vi "obs2lane2.vi"(11 "sensors inputs":dbl[][](array[numeric])=[[-2.6493086559458767, 9.313377271515247, 0.316177936945349, -1.2], [-2.6066100840450477, 9.354542103994737, 0.3157590885476819, -1.2], [-2.579340659822815, 9.43207739327695, 0.31450254335468053, -1.2], [-2.6132527619437576, 9.439068677849818, 0.5859163050429868, 1.2000000000000006], [-2.6655003955140795, 9.41719146151926, 0.4953083793337705, 0.40000000000000013], [-2.8189313467074544, 9.344249551531279, 0.5859163050429868, 1.2000000000000006], [-2.5692189092921667, 9.480018973387281, 0.5863351534406539, 1.2000000000000006], [-2.6731933264342116, 9.434269134901442, 0.5863351534406539, 1.2000000000000006], [-2.77635346299322, 9.386711660550553, 0.5863351534406539, 1.2000000000000006], [-2.7290628288714722, 9.419794899689457, 0.5865445776394874, 1.2000000000000006], [-3.035140869949269, 9.26885391372332, 0.5865445776394874, 1.2000000000000006], [-2.550914688564252, 9.509578404068655, 0.3132459981616791, -1.2], [-2.785425991035746, 9.405948172518677, 0.495587629745689, 0.40000000000000013], [-2.7463409502228373, 9.457274042188466, 0.4957970675546278, 0.40000000000000013], [-2.90576588154835, 9.392310316924437, 0.49586688015760744, 0.40000000000000013], [-2.494747129058042, 9.597974241579312, 0.5880105470313224, 1.2000000000000006], [-2.836998990617639, 9.447892074399023, 0.4039934946364334, -0.3999999999999999], [-3.1184925197733824, 9.303796817000539, 0.5880105470313224, 1.2000000000000006], [-2.970577318209098, 9.393517402151646, 0.4960763179665463, 0.40000000000000013], [-2.9699981982750367, 9.392368449256733, 0.588219971230156, 1.2000000000000006], [-3.0729809459427746, 9.340776068194645, 0.4960763179665463, 0.40000000000000013], [-3.1996655181339673, 9.27234939560896, 0.40392368203345375, -0.3999999999999999], [-3.4973819131319495, 9.096981036828707, 0.40392368203345375, -0.3999999999999999], [-2.5289827185611418, 9.605504378157487, 0.3115706045710105, -1.2], [-3.453631348161608, 9.135814142218397, 0.4038538694304742, -0.3999999999999999], [-3.2339632015510937, 9.274656811335685, 0.5886388196278232, 1.2000000000000006], [-2.483097010676977, 9.64588076688389, 0.3111517561733434, -1.2], [-2.8803018639560647, 9.47148380231442, 0.4962857557754851, 0.40000000000000013], [-2.9317308980723027, 9.444962161904348, 0.5888482438266567, 1.2000000000000006], [-2.9582194094409178, 9.433270224287725, 0.4037142442245149, -0.3999999999999999], [-3.0350382771601945, 9.392890956174119, 0.5888482438266567, 1.2000000000000006], [-2.4599617564514022, 9.665942841266034, 0.5890576680254903, 1.2000000000000006], [-3.1930649800894275, 9.320188914278454, 0.5890576680254903, 1.2000000000000006], [-3.424919733239901, 9.200023640728578, 0.4035746190185557, -0.3999999999999999], [-3.4490855593711203, 9.183917089574846, 0.5892670922243238, 1.2000000000000006], [-2.6822275888719656, 9.595825896338217, 0.49649519358442396, 0.40000000000000013], [-3.1777999006997932, 9.352779338748892, 0.40350480641557607, -0.3999999999999999], [-3.3543988506422, 9.251882705008573, 0.5894765164231575, 1.2000000000000006], [-2.4169315260491846, 9.715129108585124, 0.589685940621991, 1.2000000000000006], [-2.4440270491484113, 9.70452412526726, 0.3103140593780091, -1.2], [-2.4445036099706936, 9.705733945395902, 0.40343499381259645, -0.3999999999999999], [-2.8187951120879293, 9.544925625371082, 0.40343499381259645, -0.3999999999999999], [-2.923864294836344, 9.494810195959495, 0.40343499381259645, -0.3999999999999999], [-3.4095769435307015, 9.230983589588824, 0.589685940621991, 1.2000000000000006], [-3.032582634559555, 9.45177853739907, 0.40336518120961684, -0.3999999999999999], [-3.2893092213922506, 9.313834366383366, 0.40336518120961684, -0.3999999999999999], [-3.313999270308597, 9.298296139668594, 0.5898953648208245, 1.2000000000000006], [-2.424651387634039, 9.734980699717582, 0.4967046313933628, 0.40000000000000013], [-2.533097518783729, 9.691715080471495, 0.4967046313933628, 0.40000000000000013], [-2.6407720438905313, 9.646563404831404, 0.4967046313933628, 0.40000000000000013], [-3.4004241638790518, 9.27277469308272, 0.4032255560036576, -0.3999999999999999], [-2.6217419806033297, 9.676437047583807, 0.403155743400678, -0.3999999999999999], [-2.6755410498513874, 9.653323143325384, 0.403155743400678, -0.3999999999999999], [-2.782523848427478, 9.605691332564723, 0.403155743400678, -0.3999999999999999], [-3.072259099823128, 9.465159649093863, 0.496844256599322, 0.40000000000000013], [-3.1500774192579093, 9.424433970288224, 0.403155743400678, -0.3999999999999999], [-3.605192513867668, 9.159018691750026, 0.403155743400678, -0.3999999999999999], [-2.5981277248582337, 9.69583138333276, 0.5907330616161588, 1.2000000000000006], [-3.102875064220138, 9.460567540591395, 0.4030859307976984, -0.3999999999999999], [-3.3599181191701257, 9.319548891673922, 0.4030859307976984, -0.3999999999999999], [-3.385278626883318, 9.304833131837459, 0.49691406920230163, 0.40000000000000013], [-2.5247869108477885, 9.749066890716904, 0.40294630559173916, -0.3999999999999999], [-2.5792234787521573, 9.726796302794572, 0.40294630559173916, -0.3999999999999999], [-3.551164984637863, 9.238618668727831, 0.5913613342126596, 1.2000000000000006], [-2.394482152160173, 9.820127604989409, 0.5915707584114931, 1.2000000000000006], [-2.7494727028492556, 9.675416799445248, 0.40280668038577994, -0.3999999999999999], [-3.681670154810481, 9.169274879714472, 0.40280668038577994, -0.3999999999999999], [-2.349619394154346, 9.868922054648976, 0.5921990310079939, 1.2000000000000006], [-2.625703441413957, 9.761592003343525, 0.497402757423159, 0.40000000000000013], [-3.2137622211581482, 9.48110235361721, 0.497402757423159, 0.40000000000000013], [-3.7275762623275384, 9.185498662423365, 0.5924084552068274, 1.2000000000000006], [-2.3569997188774257, 9.88892730018629, 0.4975423826291182, 0.40000000000000013], [-3.6331178758069624, 9.258143332791025, 0.5926178794056609, 1.2000000000000006], [-3.280263464375405, 9.479130763175284, 0.4976121952320978, 0.40000000000000013], [-2.450699178158054, 9.884289629873633, 0.30675384799783845, -1.2], [-2.4511770399787394, 9.885534502477135, 0.40224817956194303, -0.3999999999999999], [-2.5345511058394776, 9.852902522117958, 0.49775182043805705, 0.40000000000000013], [-3.824786250125524, 9.17047880734031, 0.40224817956194303, -0.3999999999999999], [-2.405397050205525, 9.933526651907876, 0.3061255754013377, -1.2], [-3.4089243051435196, 9.464380504252652, 0.4979612582469959, 0.40000000000000013], [-3.56907303823246, 9.381650335067114, 0.4980310708499755, 0.40000000000000013], [-3.532949127216187, 9.438353586460368, 0.49824050865891434, 0.40000000000000013], [-3.737313762681747, 9.3103050041449, 0.5947121213939967, 1.2000000000000006], [-2.2908474536598415, 10.059979664182297, 0.595549818189331, 1.2000000000000006], [-2.3765186719612967, 10.02943138812595, 0.3044501818106692, -1.2], [-2.462262709016492, 9.999031326649108, 0.4985197590708328, 0.40000000000000013], [-3.657097646318684, 9.409803942456133, 0.4985197590708328, 0.40000000000000013], [-3.835868568229564, 9.295365230962426, 0.40148024092916723, -0.3999999999999999], [-2.3581413988349413, 10.067967806625958, 0.5961780907858316, 1.2000000000000006], [-3.877029743260587, 9.302385055789298, 0.5961780907858316, 1.2000000000000006], [-3.9331436519651666, 9.276595165706414, 0.5963875149846652, 1.2000000000000006], [-3.425151432335213, 9.616047962173518, 0.4989386346887105, 0.40000000000000013], [-2.3143719287589564, 10.127343415537375, 0.49900844729169014, 0.40000000000000013], [-3.7975482431761254, 9.403949992407117, 0.49900844729169014, 0.40000000000000013], [-3.854407472044735, 9.378948406292697, 0.49907825989466975, 0.40000000000000013], [-2.407763132093687, 10.115274836822742, 0.4008519275023507, -0.3999999999999999], [-2.468901871015975, 10.10337801061548, 0.4007821148993711, -0.3999999999999999], [-2.3890129763037065, 10.15395227178771, 0.4993575103065882, 0.40000000000000013], [-3.777898705712374, 9.487607060347795, 0.4994273229095678, 0.40000000000000013], [-4.0346920104398265, 9.315984499311078, 0.5982723327741674, 1.2000000000000006], [-4.015722357091047, 9.342912286209264, 0.40050286448745265, -0.3999999999999999], [-2.372846250599384, 10.200711102617147, 0.30109939462933205, -1.2], [-2.3833228936159903, 10.23029622982958, 0.4001538014725545, -0.3999999999999999], [-3.9666747963375277, 9.4365483588187, 0.4998461985274455, 0.40000000000000013], [-2.30100181314674, 10.278532756817912, 0.5999477263648358, 1.2000000000000006], [-4.109576508398126, 9.423930057048132, 0.5003348867483028, 0.40000000000000013], [-2.35334151682133, 10.334600032038626, 0.2985863042433292, -1.2], [-4.074608378760497, 9.48436394539886, 0.5005443245572416, 0.40000000000000013], [-2.3368079650044735, 10.384014278769136, 0.5007537623661805, 0.40000000000000013], [-2.370078405901655, 10.38320748736416, 0.39917642503083994, -0.3999999999999999], [-4.204212822255533, 9.504238162023881, 0.3988273620159418, -0.3999999999999999], [-2.2707767805352264, 10.48873231405309, 0.2960732138573263, -1.2], [-2.3200348724405737, 10.53572713543776, 0.6051833313356751, 1.2000000000000006], [-2.245779677656643, 10.622703152908741, 0.29356012347132354, -1.2], [-2.279884830624796, 10.622358187824348, 0.6066493007275101, 1.2000000000000006], [-2.358065997017253, 10.651060149761754, 0.5025688900436505, 0.40000000000000013], [-2.206922249961846, 10.718517420078616, 0.29188472988065495, -1.2], [-2.310815072326706, 10.718984235455277, 0.5029179530585486, 0.40000000000000013], [-2.250256927274077, 10.7470116403635, 0.6089529669146794, 1.2000000000000006], [-2.4078141528407944, 10.696197951674801, 0.2910470330853207, -1.2], [-2.2625570787999116, 10.786624601979373, 0.5032670160734467, 0.40000000000000013], [-2.37319268235858, 10.803936049039782, 0.3963839209116553, -0.3999999999999999], [-2.4400133449020482, 10.792431192800741, 0.3963141083086757, -0.3999999999999999], [-2.3484550625403937, 10.948347869936686, 0.3954763570729203, -0.3999999999999999], [-2.2532005442925973, 10.986565753726355, 0.6137697234878515, 1.2000000000000006], [-2.2241527610867795, 11.130722431723722, 0.6164922380726879, 1.2000000000000006], [-2.3272220554510197, 11.112000353866012, 0.3944291680282261, -0.3999999999999999], [-2.2968682826047866, 11.131657762965752, 0.5056406445747536, 0.40000000000000013], [-2.2805508875817773, 11.32421563798276, 0.5068972714283867, 0.40000000000000013], [-2.3203488195890745, 11.3333663356091, 0.39296310336565415, -0.3999999999999999], [-2.2253235316083524, 11.390402063747686, 0.6217278430435271, 1.2000000000000006], [-2.23390046248441, 11.420813566670208, 0.5074557722522236, 0.40000000000000013], [-2.315297365324197, 11.574401473618405, 0.391357413497123, -0.3999999999999999], [-2.2168668356954866, 11.63137340411444, 0.6265445996166993, 1.2000000000000006], [-2.3994033185138965, 11.600249851280598, 0.2730365519856337, -1.2], [-2.233080590823236, 11.690844769333019, 0.5092708999296937, 0.40000000000000013], [-2.3589382981537037, 11.726595493110718, 0.27073288579846444, -1.2], [-2.3008663461775223, 11.796656013544418, 0.38989134883455107, -0.3999999999999999], [-2.209460232985442, 11.892117815907735, 0.6317802045875385, 1.2000000000000006], [-2.2516708194251622, 11.903349900014954, 0.3892630354077345, -0.3999999999999999], [-2.324463966690179, 11.881746284197003, 0.26780094701479445, -1.2], [-2.2175289279374653, 11.922764866099948, 0.5108067771952451, 0.40000000000000013], [-2.2538194745555633, 11.911368790129554, 0.2675915228159609, -1.2], [-2.178403555854863, 12.077484518563601, 0.5117841536369597, 0.40000000000000013], [-2.1829008579162608, 12.095192687788384, 0.6357592643653763, 1.2000000000000006], [-2.2383426880850124, 12.155028982889158, 0.3875875329362237, -0.3999999999999999], [-2.2804615843118747, 12.317890670472249, 0.25921455486261813, -1.2], [-2.2227746224162255, 12.415062075134333, 0.2575391612719496, -1.2], [-2.186230627716147, 12.434387153701119, 0.6426702629268841, 1.2000000000000006], [-2.196164124819029, 12.474982005763925, 0.5145068451531648, 0.40000000000000013], [-2.1425536546232067, 12.599100045840768, 0.6458116259093877, 1.2000000000000006], [-2.2643337612516414, 12.581746676789589, 0.3846554036110799, -0.3999999999999999], [-2.198573038349574, 12.65771577116447, 0.2527224046987775, -1.2], [-2.1750587039156537, 12.73714405461915, 0.5162521602276552, 0.40000000000000013], [-2.238686482838199, 12.824800292270476, 0.38304971374254876, -0.3999999999999999], [-2.1747996213790666, 12.920092091405744, 0.24748679972793824, -1.2], [-2.1535345564869504, 13.01725329936264, 0.6543980180615641, 1.2000000000000006], [-2.187058282696622, 13.165406851352257, 0.519184289552799, 0.40000000000000013], [-2.0682676188644926, 13.230434114169201, 0.24162292216059827, -1.2], [-2.249455724453499, 13.24346320074072, 0.3801873970203845, -0.3999999999999999], [-2.168249294443763, 13.280340530506738, 0.2401569527687633, -1.2], [-2.1361605605328022, 13.338559010168616, 0.6608901682254047, 1.2000000000000006], [-2.1577943406236098, 13.438198159944571, 0.520999417230269, 0.40000000000000013], [-2.1011219599138715, 13.601533356858653, 0.6661257731962439, 1.2000000000000006], [-2.2400954133839512, 13.604417430165359, 0.377743955916098, -0.3999999999999999], [-2.1622288912277443, 13.672487145254262, 0.3773948929011999, -0.3999999999999999], [-2.0809447496291567, 13.728170217410458, 0.23136113641775338, -1.2], [-2.148368119037393, 13.828678025980699, 0.5236522961434944, 0.40000000000000013], [-2.1431530665836362, 14.033933863880375, 0.37495145179691336, -0.3999999999999999], [-2.106513383233814, 14.090157922222986, 0.6761781347402553, 1.2000000000000006], [-2.116678410658171, 14.141260966031997, 0.5257466742328829, 0.40000000000000013], [-2.0736923856429295, 14.42245242291376, 0.6828797091029295, 1.2000000000000006], [-2.0946138788714483, 14.532649102029193, 0.5283995531461083, 0.40000000000000013], [-2.152273017194013, 14.572484794069997, 0.3712513838389937, -0.3999999999999999], [-2.0231688076393577, 14.688270075344283, 0.5293769295878229, 0.40000000000000013], [-2.0756120529212976, 14.699000478760663, 0.37048344520621795, -0.3999999999999999], [-2.0476810196035475, 14.823824383301131, 0.6910472528574387, 1.2000000000000006], [8.784462172926562, 11.47924364037722, 0.6985865240154472, 1.2000000000000006], [8.643867253715156, 11.631338367097312, 0.6985865240154472, 1.2000000000000006], [-2.01182307782236, 15.20812065601524, 0.5329373723397832, 0.40000000000000013], [8.86867671544905, 11.41559660678595, 0.6990053724131143, 1.2000000000000006], [8.58702381954077, 11.72028699299172, 0.6990053724131143, 1.2000000000000006], [8.952448256526495, 11.35108640713428, 0.6994242208107815, 1.2000000000000006], [8.751204607664915, 11.589530329880938, 0.699633645009615, 1.2000000000000006], [-2.0698358361213067, 15.238622346987988, 0.36678337724829835, -0.3999999999999999], [8.78228318958885, 11.618259075505645, 0.5334958731636202, 0.40000000000000013], [9.066064089233228, 11.311820599800757, 0.7006807660037829, 1.2000000000000006], [8.586576710391817, 11.864672700124274, 0.7010996144014501, 1.2000000000000006], [8.904607069385332, 11.588375580628155, 0.5339845613844775, 0.40000000000000013], [8.9823118978036, 11.517019884769494, 0.5340543739874571, 0.40000000000000013], [-2.038520846959818, 15.363492520347437, 0.7021467353956179, 1.2000000000000006], [8.791223365347536, 11.769957155305526, 0.5342638117963959, 0.40000000000000013], [8.577157812432615, 12.002632694506751, 0.7029844321909522, 1.2000000000000006], [9.089521761789143, 11.471296644949536, 0.5344034370023552, 0.40000000000000013], [8.747614402156172, 11.874019031613333, 0.5345430622083145, 0.40000000000000013], [9.196614789945517, 11.42431028033962, 0.5347525000172533, 0.40000000000000013], [8.702856524966558, 11.977947480441758, 0.5348223126202329, 0.40000000000000013], [8.551902917074258, 12.126859885849031, 0.7044504015827872, 1.2000000000000006], [9.301763328727434, 11.37452391977877, 0.7052880983781215, 1.2000000000000006], [8.546058430068586, 12.272774370500398, 0.7065446435711229, 1.2000000000000006], [8.713762205484503, 12.13805016075561, 0.5356600638559883, 0.40000000000000013], [9.379898466547676, 11.440670196564861, 0.5357996890619475, 0.40000000000000013], [8.680290014842434, 12.256372289618902, 0.536078939473866, 0.40000000000000013], [-1.9947666269032363, 15.748326418663561, 0.5366374402977029, 0.40000000000000013], [5.4033137061696035, 14.702228724352713, 0.7105237033489606, 1.2000000000000006], [5.31065139179097, 14.760192151279867, 0.5369166907096213, 0.40000000000000013], [5.318145573506214, 14.776082090179019, 0.7111519759454614, 1.2000000000000006], [5.372647557345696, 14.763989846509837, 0.36287387148143985, -0.3999999999999999], [5.430433378499369, 14.758453624273042, 0.5372657537245195, 0.40000000000000013], [5.282599535397169, 14.828571261939807, 0.3627342462754806, -0.3999999999999999], [-2.0630447970868317, 15.828269580660534, 0.3627342462754806, -0.3999999999999999], [-2.0425899368277762, 16.04197255374355, 0.7161781567174671, 1.2000000000000006], [8.986023479525567, 16.697743175440838, 0.7844504455372108, 1.2000000000000006], [8.870510744967275, 16.775657498704163, 0.7844504455372108, 1.2000000000000006], [8.776249405862337, 16.886004939029128, 0.7852881423325451, 1.2000000000000006], [9.255378545456706, 16.596057732863006, 0.7859164149290457, 1.2000000000000006], [9.146441633836046, 16.684541131912827, 0.7861258391278794, 1.2000000000000006], [9.094705994581439, 16.85736482840408, 0.5628171664150587, 0.40000000000000013], [9.445245140600367, 16.620273164434607, 0.7886389295138823, 1.2000000000000006], [8.745638718171325, 17.096618222434593, 0.7886389295138823, 1.2000000000000006], [9.250822015437112, 16.835004830220694, 0.563305854635916, 0.40000000000000013], [8.898582257650931, 17.072593546817984, 0.563305854635916, 0.40000000000000013], [9.372609476756939, 16.761935663932476, 0.5633756672388956, 0.40000000000000013], [9.022240713238299, 17.00273744358763, 0.5633756672388956, 0.40000000000000013], [9.671704217358442, 16.690540187776413, 0.79261798929172, 1.2000000000000006], [8.733353836557999, 17.341528099528503, 0.7928274134905535, 1.2000000000000006], [9.575618663038583, 16.801373411419853, 0.5644228562835899, 0.40000000000000013], [8.86635551362631, 17.284293500790973, 0.5644228562835899, 0.40000000000000013], [-11.730647795102412, 15.437193920648374, 0.09942389115260453, -1.2], [-11.753961919567294, 15.46091854606451, 0.3329242648031848, -0.3999999999999999], [-2.6376199176507695, 22.880864643377365, 0.586553451428128, 0.40000000000000013], [-2.8095170709695823, 22.87690194098971, 0.5866930766340872, 0.40000000000000013], [-2.472177558679492, 22.932903386537202, 0.5867628892370669, 0.40000000000000013], [-2.1457138125258957, 23.092372962417727, 0.5876006404728222, 0.40000000000000013], [-1.975660428365826, 23.120301035359756, 0.5876704530758019, 0.40000000000000013], [-2.830488522803034, 23.021539526550544, 0.8631939442986329, 1.2000000000000006], [-2.321307029798844, 23.112624067398425, 0.5878798908847407, 0.40000000000000013], [-2.664069979468923, 23.075216022238337, 0.8638222168951337, 1.2000000000000006], [-2.4981915740055283, 23.137390254704062, 0.864659913690468, 1.2000000000000006], [-2.3314305321547493, 23.198157106933053, 0.8654976104858023, 1.2000000000000006], [-1.8217528316749911, 23.325992950774253, 0.5889968925324145, 0.40000000000000013], [-2.1768599709453524, 23.37676650480826, 0.8688483976671393, 1.2000000000000006], [-15.001217509405912, 16.7719561296704, 0.31016535623183017, -0.3999999999999999], [-15.131558329077535, 16.65366297795977, 0.31002573102587094, -0.3999999999999999], [-14.921984448489132, 16.935815146369087, 0.30981629321693205, -0.3999999999999999], [-15.241790010790758, 16.749485916960253, 0.026963118356189475, -1.2], [-15.133075455565274, 16.88861418597005, 0.0267536941573559, -1.2], [-15.017973364486107, 17.261437164441947, 0.3077917277305232, -0.3999999999999999], [9.64601974480163, 21.452115753566822, 0.5922780848724565, 0.40000000000000013], [9.496453028675626, 21.54978831901161, 0.8772253656204823, 1.2000000000000006], [9.33857931433906, 21.631972172843444, 0.8772253656204823, 1.2000000000000006], [9.17999443103193, 21.712775206793534, 0.8772253656204823, 1.2000000000000006], [-15.156829567346312, 17.1472706411717, 0.022774634379518044, -1.2], [9.377029264437805, 21.70662736414938, 0.5929762109022526, 0.40000000000000013], [9.544865059367709, 21.641804454240944, 0.5931158361082118, 0.40000000000000013], [9.710389454590258, 21.571913609233842, 0.8797384560064849, 1.2000000000000006], [-1.8772014233671248, 23.929435618135358, 0.8797384560064849, 1.2000000000000006], [9.095883042737146, 21.944626194626313, 0.8807855770006529, 1.2000000000000006], [9.271801932592034, 21.894917952170292, 0.5938139621380081, 0.40000000000000013], [-15.236180272734178, 17.461386956855613, 0.017120181011011648, -1.2], [9.194957789557106, 22.145529906980062, 0.5951404015946207, 0.40000000000000013], [5.3379716006680615, 24.14040468850077, 0.30115953044745974, -0.3999999999999999], [5.346343602955266, 24.94301298686431, 0.29571414741504976, -0.3999999999999999], [-16.03827076279453, 20.400810973707614, 0.28733663505749585, -0.3999999999999999], [-15.917453817284267, 20.56937941691859, 0.2870573846455774, -0.3999999999999999], [-15.794914133758107, 20.737124067829413, 0.28677813423365894, -0.3999999999999999], [-14.857892347507073, 21.847969012040384, 0.2851724443651278, -0.3999999999999999], [-15.023801434595246, 21.725328510394597, 0.2851026317621482, -0.3999999999999999], [-15.339589077483758, 21.460351215716504, 0.2851026317621482, -0.3999999999999999], [-15.650704132941332, 21.189903024072276, 0.2851026317621482, -0.3999999999999999], [-15.201556508849778, 21.61650958244562, 0.28489319395320933, -0.3999999999999999], [-14.728337374906722, 22.016057756865447, 0.2848233813502297, -0.3999999999999999], [-15.626945243640977, 21.4767441096572, 0.28370637970255586, -0.3999999999999999], [9.50763508171292, 26.73975570562619, 0.6252994460818146, 0.40000000000000013], [-1.4252219468434035, 28.59895493907886, 0.6255088838907534, 0.40000000000000013], [9.725543674751258, 26.692789231824694, 0.6255786964937331, 0.40000000000000013], [9.943355423856874, 26.64378657215293, 0.6258579469056516, 0.40000000000000013], [9.334114379546264, 26.89614247546073, 0.6258579469056516, 0.40000000000000013], [9.216574706656742, 27.200382540182076, 0.6275334493771623, 0.40000000000000013], [10.040081267648652, 26.868922071117122, 0.9827751618326013, 1.2000000000000006], [-1.4946609322957394, 29.821814277404098, 1.0022516123241232, 1.2000000000000006], [9.883884675811041, 31.803099088007194, 0.6592981837328874, 0.40000000000000013], [9.665449175747526, 31.97349509801759, 0.659926497159704, 0.40000000000000013], [10.174424429491456, 31.838119222564067, 0.6602057475716224, 0.40000000000000013], [10.17244090528941, 31.83259465007272, 1.0805762626878783, 1.2000000000000006], [-1.0364518801246452, 37.42334336490329, 0.6869439745128152, 0.40000000000000013], [10.026103833352638, 36.8130958059697, 0.6928780457660825, 0.40000000000000013], [9.743408822772697, 36.92812129013003, 0.6930874835750214, 0.40000000000000013], [10.347031193921643, 36.82288619877287, 1.1808904539291583, 1.2000000000000006], [-21.069030510629236, 31.45954783569295, 0.20558607696836614, -0.3999999999999999], [-21.391355310423045, 31.377757000004777, 0.20467851312963112, -0.3999999999999999], [10.4210427571751, 41.72394225688742, 0.7265975330052368, 0.40000000000000013], [10.107451026305094, 41.89078819565647, 0.7271560338290737, 0.40000000000000013], [10.474235594988285, 41.919051326913184, 1.284136583954108, 1.2000000000000006], [10.13857155297352, 42.00899223589921, 1.284136583954108, 1.2000000000000006], [10.830210018606069, 41.90102810572798, 0.7285522858886659, 0.40000000000000013], [-0.709038750028526, 57.66347671663537, 1.5846603092802805, 1.2000000000000006], [11.120605021860856, 56.96437033164037, 0.8312466248716806, 0.40000000000000013], [-0.7151980727209852, 58.133987434462625, 0.8314560626806193, 0.40000000000000013], [1.5195348183779678, 61.52869356204023, 0.04473783970333195, -0.3999999999999999], [5.073212151726797, 61.48708023724171, 0.04362083805565814, -0.3999999999999999], [11.439817695944253, 61.011847285540675, 0.8593811038724656, 0.40000000000000013], [11.689176472740309, 65.06866600393317, 0.8875155828732506, 0.40000000000000013], [14.49832831315618, 65.07219891982305, 1.7750269060199955, 1.2000000000000006], [8.818111571073048, 72.81602044955893, 1.9136657256478184, 1.2000000000000006], [12.551831810983316, 72.91253923612891, 0.9424581014182081, 0.40000000000000013], [13.768405529858791, 72.71844886386302, 1.9283254195661683, 1.2000000000000006], [1.2476421313017925, 74.97736983119862, -0.04909029870127124, -0.3999999999999999], [0.9387629168292289, 75.21210795753403, 0.9506959885698028, 0.40000000000000013], [17.77975821366545, 76.1598746565128, 2.0169118556727685, 1.2000000000000006], [47.35648972259149, 63.571420836353425, 2.052304545275642, 1.2000000000000006], [13.031972557350265, 79.3416128979354, 2.061938058421986, 1.2000000000000006], [24.83184721270082, 81.07466865802802, 2.156178947897092, 1.2000000000000006], [13.551875448365177, 86.71163580640813, 1.0385900557211387, 0.40000000000000013], [52.872675769586, 69.37798867554798, 2.2194250559448303, 1.2000000000000006], [8.915518332671137, 92.0400907270114, 1.0712623539155988, 0.40000000000000013], [9.692181670683942, 91.99867908899289, 1.0715416043275172, 0.40000000000000013], [20.71894414488982, 95.06455786989261, 2.4164932270472192, 1.2000000000000006], [19.150342204408794, 95.56882049865551, 2.4198440142285564, 1.2000000000000006], [23.490178905085354, 95.9928006820069, 2.448953977866423, 1.2000000000000006], [26.036285319817722, 95.81770414584793, 2.4592157636092677, 1.2000000000000006], [14.717578948116746, 99.12164584891, 1.1254369338277803, 0.40000000000000013], [20.65463162219833, 155.2673630873944, 3.658378726130288, 1.2000000000000006], [12.312708261276875, 191.3556263648354, 4.393457664036117, 1.2000000000000006], [14.978259637770336, 232.0240814937235, 2.048848233439155, 0.40000000000000013], [33.73593705129936, 288.53349296533526, 2.4538311433239053, 0.40000000000000013], [8.92096999050232, 17.23708913161584, 0.3356469563193898, -0.3999999999999999], [-2.5256202703736608, 22.68399055587274, 0.31491261323444397, -0.3999999999999999], [-1.8996165215080512, 23.228271875851924, 0.3116314208944021, -0.3999999999999999], [-3.0296332585078587, 23.183843349397314, 0.8671730040764709, 1.2000000000000006], [5.104128617356655, 23.236200962780366, 0.022984058578351618, -1.2], [-1.2548826959515347, 24.01715071826592, 0.01942384719818102, -1.2], [5.221948215230284, 24.444090337557157, -0.0021468452816766903, -1.2], [-2.224688830349968, 25.593404278777417, 0.9151311456093583, 1.2000000000000006], [5.209357772395169, 25.198536731676327, -0.017434811796527283, -1.2], [-1.1725915542855405, 25.874379726198075, -0.019319629586029397, -1.2], [-15.005798944565672, 21.383214801932546, -0.039005504276384995, -1.2], [-14.976356804490646, 21.66777357175441, -0.04319398825305637, -1.2], [-14.955664951264778, 21.9687081224078, -0.04780132062739484, -1.2], [9.275033221452706, 26.45651279141699, 0.277143995022472, -0.3999999999999999], [9.363878146139614, 27.271589550954324, 0.2716287993870824, -0.3999999999999999], [9.371321144452127, 28.564736959442584, 0.26318147442654893, -0.3999999999999999], [10.747513637749273, 30.43885569655537, 1.0575396008161857, 1.2000000000000006], [11.012472531760006, 30.418068389611857, 1.0592149944068543, 1.2000000000000006], [11.266285997376329, 30.367042635463775, 1.060262115401022, 1.2000000000000006], [-20.735017036098906, 31.521767273772653, 0.20663326601306034, -0.3999999999999999], [-20.49557227262787, 31.709735125755284, 0.20656345341008076, -0.3999999999999999], [10.724864676049275, 37.00446773130826, 0.6956007372822874, 0.40000000000000013], [-21.806198041420327, 31.41066071306105, 0.20272376024620187, -0.3999999999999999], [10.97816933233072, 46.72664514439962, 0.7613642092890853, 0.40000000000000013], [-33.95444016665767, 37.454440166657676, 0.11475988049188635, -0.3999999999999999], [-33.46782468155926, 38.15694699438283, 0.11364287884421248, -0.3999999999999999], [-32.258000408687934, 39.32613895725404, 0.11343344103527364, -0.3999999999999999], [-34.39923085728631, 37.30403001674005, 0.11329381582931441, -0.3999999999999999], [11.618566184124763, 57.01187131155995, 0.8322938139163747, 0.40000000000000013], [16.615400312068406, 60.50485600252477, 1.6937703168725702, 1.2000000000000006], [13.205163345895427, 64.3192947748755, 1.7536656377389712, 1.2000000000000006], [20.538690765112868, 64.00503191176435, 1.7884300547453438, 1.2000000000000006], [13.026046392769018, 79.30712465157343, 0.9869985421192027, 0.40000000000000013], [27.29899080749756, 81.67230442986731, 2.1844512147396244, 1.2000000000000006], [33.69042505267091, 80.06731529671714, 2.2022522716404778, 1.2000000000000006], [29.157427120978678, 82.5346645544511, 2.2146082993716583, 1.2000000000000006], [27.17382907061827, 93.78874887901951, 2.425079619199396, 1.2000000000000006], [34.761055666251615, 92.88790635480824, 2.4590063394104344, 1.2000000000000006], [-2.729118001525531, 22.918683596868465, 0.31309748555697403, -0.3999999999999999], [9.124522914489708, 21.80096170236561, 0.3072332269066863, -0.3999999999999999], [-1.5170192378515415, 28.303045293335575, 0.2765156815956554, -0.3999999999999999], [-1.3900091234452605, 30.022954081648294, 0.2645777264861412, -0.3999999999999999], [4.034616118215339, 61.19769858054814, 0.04620390436590388, -0.3999999999999999], [26.121526235859253, 82.71602090547535, 2.197226090868472, 1.2000000000000006]]) -> ()   [LabVIEW 2012]
uses:
  G_SEN.vi
  <vilib>/Analysis/Matrix/Numeric/Conversions/Array To Matrix - RA2.vi
  <vilib>/Analysis/baseanly.llb/Real Inverse Matrix.vi
  <vilib>/Analysis/baseanly.llb/A x Vector.vi
  <vilib>/Analysis/Matrix/NI_Matrix.lvlib
  <vilib>/Analysis/NI_AALBase.lvlib
panel:
  out "lanes 2":dbl[][](array[numeric])
  out "lane_seed":dbl[][](array[numeric])
  in  "Numeric":dbl=0.8
  in  "lane num":i32=6
  in  "order":i32=2 min=0 max=2 step=1
  out "lane lenght":dbl[](array[numeric])
  out "lane count":i16[](array[numeric])
  out "time":u32
  out "lanes":dbl[][](array[numeric])
  out "lane_x":dbl[](array[numeric])
  out "sensors":dbl[][](array[numeric])=[[-2.6493086559458767, 9.313377271515247, 0.316177936945349, -1.2], [-2.6066100840450477, 9.354542103994737, 0.3157590885476819, -1.2], [-2.579340659822815, 9.43207739327695, 0.31450254335468053, -1.2], [-2.6132527619437576, 9.439068677849818, 0.5859163050429868, 1.2000000000000006], [-2.6655003955140795, 9.41719146151926, 0.4953083793337705, 0.40000000000000013], [-2.8189313467074544, 9.344249551531279, 0.5859163050429868, 1.2000000000000006], [-2.5692189092921667, 9.480018973387281, 0.5863351534406539, 1.2000000000000006], [-2.6731933264342116, 9.434269134901442, 0.5863351534406539, 1.2000000000000006], [-2.77635346299322, 9.386711660550553, 0.5863351534406539, 1.2000000000000006], [-2.7290628288714722, 9.419794899689457, 0.5865445776394874, 1.2000000000000006], [-3.035140869949269, 9.26885391372332, 0.5865445776394874, 1.2000000000000006], [-2.550914688564252, 9.509578404068655, 0.3132459981616791, -1.2], [-2.785425991035746, 9.405948172518677, 0.495587629745689, 0.40000000000000013], [-2.7463409502228373, 9.457274042188466, 0.4957970675546278, 0.40000000000000013], [-2.90576588154835, 9.392310316924437, 0.49586688015760744, 0.40000000000000013], [-2.494747129058042, 9.597974241579312, 0.5880105470313224, 1.2000000000000006], [-2.836998990617639, 9.447892074399023, 0.4039934946364334, -0.3999999999999999], [-3.1184925197733824, 9.303796817000539, 0.5880105470313224, 1.2000000000000006], [-2.970577318209098, 9.393517402151646, 0.4960763179665463, 0.40000000000000013], [-2.9699981982750367, 9.392368449256733, 0.588219971230156, 1.2000000000000006], [-3.0729809459427746, 9.340776068194645, 0.4960763179665463, 0.40000000000000013], [-3.1996655181339673, 9.27234939560896, 0.40392368203345375, -0.3999999999999999], [-3.4973819131319495, 9.096981036828707, 0.40392368203345375, -0.3999999999999999], [-2.5289827185611418, 9.605504378157487, 0.3115706045710105, -1.2], [-3.453631348161608, 9.135814142218397, 0.4038538694304742, -0.3999999999999999], [-3.2339632015510937, 9.274656811335685, 0.5886388196278232, 1.2000000000000006], [-2.483097010676977, 9.64588076688389, 0.3111517561733434, -1.2], [-2.8803018639560647, 9.47148380231442, 0.4962857557754851, 0.40000000000000013], [-2.9317308980723027, 9.444962161904348, 0.5888482438266567, 1.2000000000000006], [-2.9582194094409178, 9.433270224287725, 0.4037142442245149, -0.3999999999999999], [-3.0350382771601945, 9.392890956174119, 0.5888482438266567, 1.2000000000000006], [-2.4599617564514022, 9.665942841266034, 0.5890576680254903, 1.2000000000000006], [-3.1930649800894275, 9.320188914278454, 0.5890576680254903, 1.2000000000000006], [-3.424919733239901, 9.200023640728578, 0.4035746190185557, -0.3999999999999999], [-3.4490855593711203, 9.183917089574846, 0.5892670922243238, 1.2000000000000006], [-2.6822275888719656, 9.595825896338217, 0.49649519358442396, 0.40000000000000013], [-3.1777999006997932, 9.352779338748892, 0.40350480641557607, -0.3999999999999999], [-3.3543988506422, 9.251882705008573, 0.5894765164231575, 1.2000000000000006], [-2.4169315260491846, 9.715129108585124, 0.589685940621991, 1.2000000000000006], [-2.4440270491484113, 9.70452412526726, 0.3103140593780091, -1.2], [-2.4445036099706936, 9.705733945395902, 0.40343499381259645, -0.3999999999999999], [-2.8187951120879293, 9.544925625371082, 0.40343499381259645, -0.3999999999999999], [-2.923864294836344, 9.494810195959495, 0.40343499381259645, -0.3999999999999999], [-3.4095769435307015, 9.230983589588824, 0.589685940621991, 1.2000000000000006], [-3.032582634559555, 9.45177853739907, 0.40336518120961684, -0.3999999999999999], [-3.2893092213922506, 9.313834366383366, 0.40336518120961684, -0.3999999999999999], [-3.313999270308597, 9.298296139668594, 0.5898953648208245, 1.2000000000000006], [-2.424651387634039, 9.734980699717582, 0.4967046313933628, 0.40000000000000013], [-2.533097518783729, 9.691715080471495, 0.4967046313933628, 0.40000000000000013], [-2.6407720438905313, 9.646563404831404, 0.4967046313933628, 0.40000000000000013], [-3.4004241638790518, 9.27277469308272, 0.4032255560036576, -0.3999999999999999], [-2.6217419806033297, 9.676437047583807, 0.403155743400678, -0.3999999999999999], [-2.6755410498513874, 9.653323143325384, 0.403155743400678, -0.3999999999999999], [-2.782523848427478, 9.605691332564723, 0.403155743400678, -0.3999999999999999], [-3.072259099823128, 9.465159649093863, 0.496844256599322, 0.40000000000000013], [-3.1500774192579093, 9.424433970288224, 0.403155743400678, -0.3999999999999999], [-3.605192513867668, 9.159018691750026, 0.403155743400678, -0.3999999999999999], [-2.5981277248582337, 9.69583138333276, 0.5907330616161588, 1.2000000000000006], [-3.102875064220138, 9.460567540591395, 0.4030859307976984, -0.3999999999999999], [-3.3599181191701257, 9.319548891673922, 0.4030859307976984, -0.3999999999999999], [-3.385278626883318, 9.304833131837459, 0.49691406920230163, 0.40000000000000013], [-2.5247869108477885, 9.749066890716904, 0.40294630559173916, -0.3999999999999999], [-2.5792234787521573, 9.726796302794572, 0.40294630559173916, -0.3999999999999999], [-3.551164984637863, 9.238618668727831, 0.5913613342126596, 1.2000000000000006], [-2.394482152160173, 9.820127604989409, 0.5915707584114931, 1.2000000000000006], [-2.7494727028492556, 9.675416799445248, 0.40280668038577994, -0.3999999999999999], [-3.681670154810481, 9.169274879714472, 0.40280668038577994, -0.3999999999999999], [-2.349619394154346, 9.868922054648976, 0.5921990310079939, 1.2000000000000006], [-2.625703441413957, 9.761592003343525, 0.497402757423159, 0.40000000000000013], [-3.2137622211581482, 9.48110235361721, 0.497402757423159, 0.40000000000000013], [-3.7275762623275384, 9.185498662423365, 0.5924084552068274, 1.2000000000000006], [-2.3569997188774257, 9.88892730018629, 0.4975423826291182, 0.40000000000000013], [-3.6331178758069624, 9.258143332791025, 0.5926178794056609, 1.2000000000000006], [-3.280263464375405, 9.479130763175284, 0.4976121952320978, 0.40000000000000013], [-2.450699178158054, 9.884289629873633, 0.30675384799783845, -1.2], [-2.4511770399787394, 9.885534502477135, 0.40224817956194303, -0.3999999999999999], [-2.5345511058394776, 9.852902522117958, 0.49775182043805705, 0.40000000000000013], [-3.824786250125524, 9.17047880734031, 0.40224817956194303, -0.3999999999999999], [-2.405397050205525, 9.933526651907876, 0.3061255754013377, -1.2], [-3.4089243051435196, 9.464380504252652, 0.4979612582469959, 0.40000000000000013], [-3.56907303823246, 9.381650335067114, 0.4980310708499755, 0.40000000000000013], [-3.532949127216187, 9.438353586460368, 0.49824050865891434, 0.40000000000000013], [-3.737313762681747, 9.3103050041449, 0.5947121213939967, 1.2000000000000006], [-2.2908474536598415, 10.059979664182297, 0.595549818189331, 1.2000000000000006], [-2.3765186719612967, 10.02943138812595, 0.3044501818106692, -1.2], [-2.462262709016492, 9.999031326649108, 0.4985197590708328, 0.40000000000000013], [-3.657097646318684, 9.409803942456133, 0.4985197590708328, 0.40000000000000013], [-3.835868568229564, 9.295365230962426, 0.40148024092916723, -0.3999999999999999], [-2.3581413988349413, 10.067967806625958, 0.5961780907858316, 1.2000000000000006], [-3.877029743260587, 9.302385055789298, 0.5961780907858316, 1.2000000000000006], [-3.9331436519651666, 9.276595165706414, 0.5963875149846652, 1.2000000000000006], [-3.425151432335213, 9.616047962173518, 0.4989386346887105, 0.40000000000000013], [-2.3143719287589564, 10.127343415537375, 0.49900844729169014, 0.40000000000000013], [-3.7975482431761254, 9.403949992407117, 0.49900844729169014, 0.40000000000000013], [-3.854407472044735, 9.378948406292697, 0.49907825989466975, 0.40000000000000013], [-2.407763132093687, 10.115274836822742, 0.4008519275023507, -0.3999999999999999], [-2.468901871015975, 10.10337801061548, 0.4007821148993711, -0.3999999999999999], [-2.3890129763037065, 10.15395227178771, 0.4993575103065882, 0.40000000000000013], [-3.777898705712374, 9.487607060347795, 0.4994273229095678, 0.40000000000000013], [-4.0346920104398265, 9.315984499311078, 0.5982723327741674, 1.2000000000000006], [-4.015722357091047, 9.342912286209264, 0.40050286448745265, -0.3999999999999999], [-2.372846250599384, 10.200711102617147, 0.30109939462933205, -1.2], [-2.3833228936159903, 10.23029622982958, 0.4001538014725545, -0.3999999999999999], [-3.9666747963375277, 9.4365483588187, 0.4998461985274455, 0.40000000000000013], [-2.30100181314674, 10.278532756817912, 0.5999477263648358, 1.2000000000000006], [-4.109576508398126, 9.423930057048132, 0.5003348867483028, 0.40000000000000013], [-2.35334151682133, 10.334600032038626, 0.2985863042433292, -1.2], [-4.074608378760497, 9.48436394539886, 0.5005443245572416, 0.40000000000000013], [-2.3368079650044735, 10.384014278769136, 0.5007537623661805, 0.40000000000000013], [-2.370078405901655, 10.38320748736416, 0.39917642503083994, -0.3999999999999999], [-4.204212822255533, 9.504238162023881, 0.3988273620159418, -0.3999999999999999], [-2.2707767805352264, 10.48873231405309, 0.2960732138573263, -1.2], [-2.3200348724405737, 10.53572713543776, 0.6051833313356751, 1.2000000000000006], [-2.245779677656643, 10.622703152908741, 0.29356012347132354, -1.2], [-2.279884830624796, 10.622358187824348, 0.6066493007275101, 1.2000000000000006], [-2.358065997017253, 10.651060149761754, 0.5025688900436505, 0.40000000000000013], [-2.206922249961846, 10.718517420078616, 0.29188472988065495, -1.2], [-2.310815072326706, 10.718984235455277, 0.5029179530585486, 0.40000000000000013], [-2.250256927274077, 10.7470116403635, 0.6089529669146794, 1.2000000000000006], [-2.4078141528407944, 10.696197951674801, 0.2910470330853207, -1.2], [-2.2625570787999116, 10.786624601979373, 0.5032670160734467, 0.40000000000000013], [-2.37319268235858, 10.803936049039782, 0.3963839209116553, -0.3999999999999999], [-2.4400133449020482, 10.792431192800741, 0.3963141083086757, -0.3999999999999999], [-2.3484550625403937, 10.948347869936686, 0.3954763570729203, -0.3999999999999999], [-2.2532005442925973, 10.986565753726355, 0.6137697234878515, 1.2000000000000006], [-2.2241527610867795, 11.130722431723722, 0.6164922380726879, 1.2000000000000006], [-2.3272220554510197, 11.112000353866012, 0.3944291680282261, -0.3999999999999999], [-2.2968682826047866, 11.131657762965752, 0.5056406445747536, 0.40000000000000013], [-2.2805508875817773, 11.32421563798276, 0.5068972714283867, 0.40000000000000013], [-2.3203488195890745, 11.3333663356091, 0.39296310336565415, -0.3999999999999999], [-2.2253235316083524, 11.390402063747686, 0.6217278430435271, 1.2000000000000006], [-2.23390046248441, 11.420813566670208, 0.5074557722522236, 0.40000000000000013], [-2.315297365324197, 11.574401473618405, 0.391357413497123, -0.3999999999999999], [-2.2168668356954866, 11.63137340411444, 0.6265445996166993, 1.2000000000000006], [-2.3994033185138965, 11.600249851280598, 0.2730365519856337, -1.2], [-2.233080590823236, 11.690844769333019, 0.5092708999296937, 0.40000000000000013], [-2.3589382981537037, 11.726595493110718, 0.27073288579846444, -1.2], [-2.3008663461775223, 11.796656013544418, 0.38989134883455107, -0.3999999999999999], [-2.209460232985442, 11.892117815907735, 0.6317802045875385, 1.2000000000000006], [-2.2516708194251622, 11.903349900014954, 0.3892630354077345, -0.3999999999999999], [-2.324463966690179, 11.881746284197003, 0.26780094701479445, -1.2], [-2.2175289279374653, 11.922764866099948, 0.5108067771952451, 0.40000000000000013], [-2.2538194745555633, 11.911368790129554, 0.2675915228159609, -1.2], [-2.178403555854863, 12.077484518563601, 0.5117841536369597, 0.40000000000000013], [-2.1829008579162608, 12.095192687788384, 0.6357592643653763, 1.2000000000000006], [-2.2383426880850124, 12.155028982889158, 0.3875875329362237, -0.3999999999999999], [-2.2804615843118747, 12.317890670472249, 0.25921455486261813, -1.2], [-2.2227746224162255, 12.415062075134333, 0.2575391612719496, -1.2], [-2.186230627716147, 12.434387153701119, 0.6426702629268841, 1.2000000000000006], [-2.196164124819029, 12.474982005763925, 0.5145068451531648, 0.40000000000000013], [-2.1425536546232067, 12.599100045840768, 0.6458116259093877, 1.2000000000000006], [-2.2643337612516414, 12.581746676789589, 0.3846554036110799, -0.3999999999999999], [-2.198573038349574, 12.65771577116447, 0.2527224046987775, -1.2], [-2.1750587039156537, 12.73714405461915, 0.5162521602276552, 0.40000000000000013], [-2.238686482838199, 12.824800292270476, 0.38304971374254876, -0.3999999999999999], [-2.1747996213790666, 12.920092091405744, 0.24748679972793824, -1.2], [-2.1535345564869504, 13.01725329936264, 0.6543980180615641, 1.2000000000000006], [-2.187058282696622, 13.165406851352257, 0.519184289552799, 0.40000000000000013], [-2.0682676188644926, 13.230434114169201, 0.24162292216059827, -1.2], [-2.249455724453499, 13.24346320074072, 0.3801873970203845, -0.3999999999999999], [-2.168249294443763, 13.280340530506738, 0.2401569527687633, -1.2], [-2.1361605605328022, 13.338559010168616, 0.6608901682254047, 1.2000000000000006], [-2.1577943406236098, 13.438198159944571, 0.520999417230269, 0.40000000000000013], [-2.1011219599138715, 13.601533356858653, 0.6661257731962439, 1.2000000000000006], [-2.2400954133839512, 13.604417430165359, 0.377743955916098, -0.3999999999999999], [-2.1622288912277443, 13.672487145254262, 0.3773948929011999, -0.3999999999999999], [-2.0809447496291567, 13.728170217410458, 0.23136113641775338, -1.2], [-2.148368119037393, 13.828678025980699, 0.5236522961434944, 0.40000000000000013], [-2.1431530665836362, 14.033933863880375, 0.37495145179691336, -0.3999999999999999], [-2.106513383233814, 14.090157922222986, 0.6761781347402553, 1.2000000000000006], [-2.116678410658171, 14.141260966031997, 0.5257466742328829, 0.40000000000000013], [-2.0736923856429295, 14.42245242291376, 0.6828797091029295, 1.2000000000000006], [-2.0946138788714483, 14.532649102029193, 0.5283995531461083, 0.40000000000000013], [-2.152273017194013, 14.572484794069997, 0.3712513838389937, -0.3999999999999999], [-2.0231688076393577, 14.688270075344283, 0.5293769295878229, 0.40000000000000013], [-2.0756120529212976, 14.699000478760663, 0.37048344520621795, -0.3999999999999999], [-2.0476810196035475, 14.823824383301131, 0.6910472528574387, 1.2000000000000006], [8.784462172926562, 11.47924364037722, 0.6985865240154472, 1.2000000000000006], [8.643867253715156, 11.631338367097312, 0.6985865240154472, 1.2000000000000006], [-2.01182307782236, 15.20812065601524, 0.5329373723397832, 0.40000000000000013], [8.86867671544905, 11.41559660678595, 0.6990053724131143, 1.2000000000000006], [8.58702381954077, 11.72028699299172, 0.6990053724131143, 1.2000000000000006], [8.952448256526495, 11.35108640713428, 0.6994242208107815, 1.2000000000000006], [8.751204607664915, 11.589530329880938, 0.699633645009615, 1.2000000000000006], [-2.0698358361213067, 15.238622346987988, 0.36678337724829835, -0.3999999999999999], [8.78228318958885, 11.618259075505645, 0.5334958731636202, 0.40000000000000013], [9.066064089233228, 11.311820599800757, 0.7006807660037829, 1.2000000000000006], [8.586576710391817, 11.864672700124274, 0.7010996144014501, 1.2000000000000006], [8.904607069385332, 11.588375580628155, 0.5339845613844775, 0.40000000000000013], [8.9823118978036, 11.517019884769494, 0.5340543739874571, 0.40000000000000013], [-2.038520846959818, 15.363492520347437, 0.7021467353956179, 1.2000000000000006], [8.791223365347536, 11.769957155305526, 0.5342638117963959, 0.40000000000000013], [8.577157812432615, 12.002632694506751, 0.7029844321909522, 1.2000000000000006], [9.089521761789143, 11.471296644949536, 0.5344034370023552, 0.40000000000000013], [8.747614402156172, 11.874019031613333, 0.5345430622083145, 0.40000000000000013], [9.196614789945517, 11.42431028033962, 0.5347525000172533, 0.40000000000000013], [8.702856524966558, 11.977947480441758, 0.5348223126202329, 0.40000000000000013], [8.551902917074258, 12.126859885849031, 0.7044504015827872, 1.2000000000000006], [9.301763328727434, 11.37452391977877, 0.7052880983781215, 1.2000000000000006], [8.546058430068586, 12.272774370500398, 0.7065446435711229, 1.2000000000000006], [8.713762205484503, 12.13805016075561, 0.5356600638559883, 0.40000000000000013], [9.379898466547676, 11.440670196564861, 0.5357996890619475, 0.40000000000000013], [8.680290014842434, 12.256372289618902, 0.536078939473866, 0.40000000000000013], [-1.9947666269032363, 15.748326418663561, 0.5366374402977029, 0.40000000000000013], [5.4033137061696035, 14.702228724352713, 0.7105237033489606, 1.2000000000000006], [5.31065139179097, 14.760192151279867, 0.5369166907096213, 0.40000000000000013], [5.318145573506214, 14.776082090179019, 0.7111519759454614, 1.2000000000000006], [5.372647557345696, 14.763989846509837, 0.36287387148143985, -0.3999999999999999], [5.430433378499369, 14.758453624273042, 0.5372657537245195, 0.40000000000000013], [5.282599535397169, 14.828571261939807, 0.3627342462754806, -0.3999999999999999], [-2.0630447970868317, 15.828269580660534, 0.3627342462754806, -0.3999999999999999], [-2.0425899368277762, 16.04197255374355, 0.7161781567174671, 1.2000000000000006], [8.986023479525567, 16.697743175440838, 0.7844504455372108, 1.2000000000000006], [8.870510744967275, 16.775657498704163, 0.7844504455372108, 1.2000000000000006], [8.776249405862337, 16.886004939029128, 0.7852881423325451, 1.2000000000000006], [9.255378545456706, 16.596057732863006, 0.7859164149290457, 1.2000000000000006], [9.146441633836046, 16.684541131912827, 0.7861258391278794, 1.2000000000000006], [9.094705994581439, 16.85736482840408, 0.5628171664150587, 0.40000000000000013], [9.445245140600367, 16.620273164434607, 0.7886389295138823, 1.2000000000000006], [8.745638718171325, 17.096618222434593, 0.7886389295138823, 1.2000000000000006], [9.250822015437112, 16.835004830220694, 0.563305854635916, 0.40000000000000013], [8.898582257650931, 17.072593546817984, 0.563305854635916, 0.40000000000000013], [9.372609476756939, 16.761935663932476, 0.5633756672388956, 0.40000000000000013], [9.022240713238299, 17.00273744358763, 0.5633756672388956, 0.40000000000000013], [9.671704217358442, 16.690540187776413, 0.79261798929172, 1.2000000000000006], [8.733353836557999, 17.341528099528503, 0.7928274134905535, 1.2000000000000006], [9.575618663038583, 16.801373411419853, 0.5644228562835899, 0.40000000000000013], [8.86635551362631, 17.284293500790973, 0.5644228562835899, 0.40000000000000013], [-11.730647795102412, 15.437193920648374, 0.09942389115260453, -1.2], [-11.753961919567294, 15.46091854606451, 0.3329242648031848, -0.3999999999999999], [-2.6376199176507695, 22.880864643377365, 0.586553451428128, 0.40000000000000013], [-2.8095170709695823, 22.87690194098971, 0.5866930766340872, 0.40000000000000013], [-2.472177558679492, 22.932903386537202, 0.5867628892370669, 0.40000000000000013], [-2.1457138125258957, 23.092372962417727, 0.5876006404728222, 0.40000000000000013], [-1.975660428365826, 23.120301035359756, 0.5876704530758019, 0.40000000000000013], [-2.830488522803034, 23.021539526550544, 0.8631939442986329, 1.2000000000000006], [-2.321307029798844, 23.112624067398425, 0.5878798908847407, 0.40000000000000013], [-2.664069979468923, 23.075216022238337, 0.8638222168951337, 1.2000000000000006], [-2.4981915740055283, 23.137390254704062, 0.864659913690468, 1.2000000000000006], [-2.3314305321547493, 23.198157106933053, 0.8654976104858023, 1.2000000000000006], [-1.8217528316749911, 23.325992950774253, 0.5889968925324145, 0.40000000000000013], [-2.1768599709453524, 23.37676650480826, 0.8688483976671393, 1.2000000000000006], [-15.001217509405912, 16.7719561296704, 0.31016535623183017, -0.3999999999999999], [-15.131558329077535, 16.65366297795977, 0.31002573102587094, -0.3999999999999999], [-14.921984448489132, 16.935815146369087, 0.30981629321693205, -0.3999999999999999], [-15.241790010790758, 16.749485916960253, 0.026963118356189475, -1.2], [-15.133075455565274, 16.88861418597005, 0.0267536941573559, -1.2], [-15.017973364486107, 17.261437164441947, 0.3077917277305232, -0.3999999999999999], [9.64601974480163, 21.452115753566822, 0.5922780848724565, 0.40000000000000013], [9.496453028675626, 21.54978831901161, 0.8772253656204823, 1.2000000000000006], [9.33857931433906, 21.631972172843444, 0.8772253656204823, 1.2000000000000006], [9.17999443103193, 21.712775206793534, 0.8772253656204823, 1.2000000000000006], [-15.156829567346312, 17.1472706411717, 0.022774634379518044, -1.2], [9.377029264437805, 21.70662736414938, 0.5929762109022526, 0.40000000000000013], [9.544865059367709, 21.641804454240944, 0.5931158361082118, 0.40000000000000013], [9.710389454590258, 21.571913609233842, 0.8797384560064849, 1.2000000000000006], [-1.8772014233671248, 23.929435618135358, 0.8797384560064849, 1.2000000000000006], [9.095883042737146, 21.944626194626313, 0.8807855770006529, 1.2000000000000006], [9.271801932592034, 21.894917952170292, 0.5938139621380081, 0.40000000000000013], [-15.236180272734178, 17.461386956855613, 0.017120181011011648, -1.2], [9.194957789557106, 22.145529906980062, 0.5951404015946207, 0.40000000000000013], [5.3379716006680615, 24.14040468850077, 0.30115953044745974, -0.3999999999999999], [5.346343602955266, 24.94301298686431, 0.29571414741504976, -0.3999999999999999], [-16.03827076279453, 20.400810973707614, 0.28733663505749585, -0.3999999999999999], [-15.917453817284267, 20.56937941691859, 0.2870573846455774, -0.3999999999999999], [-15.794914133758107, 20.737124067829413, 0.28677813423365894, -0.3999999999999999], [-14.857892347507073, 21.847969012040384, 0.2851724443651278, -0.3999999999999999], [-15.023801434595246, 21.725328510394597, 0.2851026317621482, -0.3999999999999999], [-15.339589077483758, 21.460351215716504, 0.2851026317621482, -0.3999999999999999], [-15.650704132941332, 21.189903024072276, 0.2851026317621482, -0.3999999999999999], [-15.201556508849778, 21.61650958244562, 0.28489319395320933, -0.3999999999999999], [-14.728337374906722, 22.016057756865447, 0.2848233813502297, -0.3999999999999999], [-15.626945243640977, 21.4767441096572, 0.28370637970255586, -0.3999999999999999], [9.50763508171292, 26.73975570562619, 0.6252994460818146, 0.40000000000000013], [-1.4252219468434035, 28.59895493907886, 0.6255088838907534, 0.40000000000000013], [9.725543674751258, 26.692789231824694, 0.6255786964937331, 0.40000000000000013], [9.943355423856874, 26.64378657215293, 0.6258579469056516, 0.40000000000000013], [9.334114379546264, 26.89614247546073, 0.6258579469056516, 0.40000000000000013], [9.216574706656742, 27.200382540182076, 0.6275334493771623, 0.40000000000000013], [10.040081267648652, 26.868922071117122, 0.9827751618326013, 1.2000000000000006], [-1.4946609322957394, 29.821814277404098, 1.0022516123241232, 1.2000000000000006], [9.883884675811041, 31.803099088007194, 0.6592981837328874, 0.40000000000000013], [9.665449175747526, 31.97349509801759, 0.659926497159704, 0.40000000000000013], [10.174424429491456, 31.838119222564067, 0.6602057475716224, 0.40000000000000013], [10.17244090528941, 31.83259465007272, 1.0805762626878783, 1.2000000000000006], [-1.0364518801246452, 37.42334336490329, 0.6869439745128152, 0.40000000000000013], [10.026103833352638, 36.8130958059697, 0.6928780457660825, 0.40000000000000013], [9.743408822772697, 36.92812129013003, 0.6930874835750214, 0.40000000000000013], [10.347031193921643, 36.82288619877287, 1.1808904539291583, 1.2000000000000006], [-21.069030510629236, 31.45954783569295, 0.20558607696836614, -0.3999999999999999], [-21.391355310423045, 31.377757000004777, 0.20467851312963112, -0.3999999999999999], [10.4210427571751, 41.72394225688742, 0.7265975330052368, 0.40000000000000013], [10.107451026305094, 41.89078819565647, 0.7271560338290737, 0.40000000000000013], [10.474235594988285, 41.919051326913184, 1.284136583954108, 1.2000000000000006], [10.13857155297352, 42.00899223589921, 1.284136583954108, 1.2000000000000006], [10.830210018606069, 41.90102810572798, 0.7285522858886659, 0.40000000000000013], [-0.709038750028526, 57.66347671663537, 1.5846603092802805, 1.2000000000000006], [11.120605021860856, 56.96437033164037, 0.8312466248716806, 0.40000000000000013], [-0.7151980727209852, 58.133987434462625, 0.8314560626806193, 0.40000000000000013], [1.5195348183779678, 61.52869356204023, 0.04473783970333195, -0.3999999999999999], [5.073212151726797, 61.48708023724171, 0.04362083805565814, -0.3999999999999999], [11.439817695944253, 61.011847285540675, 0.8593811038724656, 0.40000000000000013], [11.689176472740309, 65.06866600393317, 0.8875155828732506, 0.40000000000000013], [14.49832831315618, 65.07219891982305, 1.7750269060199955, 1.2000000000000006], [8.818111571073048, 72.81602044955893, 1.9136657256478184, 1.2000000000000006], [12.551831810983316, 72.91253923612891, 0.9424581014182081, 0.40000000000000013], [13.768405529858791, 72.71844886386302, 1.9283254195661683, 1.2000000000000006], [1.2476421313017925, 74.97736983119862, -0.04909029870127124, -0.3999999999999999], [0.9387629168292289, 75.21210795753403, 0.9506959885698028, 0.40000000000000013], [17.77975821366545, 76.1598746565128, 2.0169118556727685, 1.2000000000000006], [47.35648972259149, 63.571420836353425, 2.052304545275642, 1.2000000000000006], [13.031972557350265, 79.3416128979354, 2.061938058421986, 1.2000000000000006], [24.83184721270082, 81.07466865802802, 2.156178947897092, 1.2000000000000006], [13.551875448365177, 86.71163580640813, 1.0385900557211387, 0.40000000000000013], [52.872675769586, 69.37798867554798, 2.2194250559448303, 1.2000000000000006], [8.915518332671137, 92.0400907270114, 1.0712623539155988, 0.40000000000000013], [9.692181670683942, 91.99867908899289, 1.0715416043275172, 0.40000000000000013], [20.71894414488982, 95.06455786989261, 2.4164932270472192, 1.2000000000000006], [19.150342204408794, 95.56882049865551, 2.4198440142285564, 1.2000000000000006], [23.490178905085354, 95.9928006820069, 2.448953977866423, 1.2000000000000006], [26.036285319817722, 95.81770414584793, 2.4592157636092677, 1.2000000000000006], [14.717578948116746, 99.12164584891, 1.1254369338277803, 0.40000000000000013], [20.65463162219833, 155.2673630873944, 3.658378726130288, 1.2000000000000006], [12.312708261276875, 191.3556263648354, 4.393457664036117, 1.2000000000000006], [14.978259637770336, 232.0240814937235, 2.048848233439155, 0.40000000000000013], [33.73593705129936, 288.53349296533526, 2.4538311433239053, 0.40000000000000013], [8.92096999050232, 17.23708913161584, 0.3356469563193898, -0.3999999999999999], [-2.5256202703736608, 22.68399055587274, 0.31491261323444397, -0.3999999999999999], [-1.8996165215080512, 23.228271875851924, 0.3116314208944021, -0.3999999999999999], [-3.0296332585078587, 23.183843349397314, 0.8671730040764709, 1.2000000000000006], [5.104128617356655, 23.236200962780366, 0.022984058578351618, -1.2], [-1.2548826959515347, 24.01715071826592, 0.01942384719818102, -1.2], [5.221948215230284, 24.444090337557157, -0.0021468452816766903, -1.2], [-2.224688830349968, 25.593404278777417, 0.9151311456093583, 1.2000000000000006], [5.209357772395169, 25.198536731676327, -0.017434811796527283, -1.2], [-1.1725915542855405, 25.874379726198075, -0.019319629586029397, -1.2], [-15.005798944565672, 21.383214801932546, -0.039005504276384995, -1.2], [-14.976356804490646, 21.66777357175441, -0.04319398825305637, -1.2], [-14.955664951264778, 21.9687081224078, -0.04780132062739484, -1.2], [9.275033221452706, 26.45651279141699, 0.277143995022472, -0.3999999999999999], [9.363878146139614, 27.271589550954324, 0.2716287993870824, -0.3999999999999999], [9.371321144452127, 28.564736959442584, 0.26318147442654893, -0.3999999999999999], [10.747513637749273, 30.43885569655537, 1.0575396008161857, 1.2000000000000006], [11.012472531760006, 30.418068389611857, 1.0592149944068543, 1.2000000000000006], [11.266285997376329, 30.367042635463775, 1.060262115401022, 1.2000000000000006], [-20.735017036098906, 31.521767273772653, 0.20663326601306034, -0.3999999999999999], [-20.49557227262787, 31.709735125755284, 0.20656345341008076, -0.3999999999999999], [10.724864676049275, 37.00446773130826, 0.6956007372822874, 0.40000000000000013], [-21.806198041420327, 31.41066071306105, 0.20272376024620187, -0.3999999999999999], [10.97816933233072, 46.72664514439962, 0.7613642092890853, 0.40000000000000013], [-33.95444016665767, 37.454440166657676, 0.11475988049188635, -0.3999999999999999], [-33.46782468155926, 38.15694699438283, 0.11364287884421248, -0.3999999999999999], [-32.258000408687934, 39.32613895725404, 0.11343344103527364, -0.3999999999999999], [-34.39923085728631, 37.30403001674005, 0.11329381582931441, -0.3999999999999999], [11.618566184124763, 57.01187131155995, 0.8322938139163747, 0.40000000000000013], [16.615400312068406, 60.50485600252477, 1.6937703168725702, 1.2000000000000006], [13.205163345895427, 64.3192947748755, 1.7536656377389712, 1.2000000000000006], [20.538690765112868, 64.00503191176435, 1.7884300547453438, 1.2000000000000006], [13.026046392769018, 79.30712465157343, 0.9869985421192027, 0.40000000000000013], [27.29899080749756, 81.67230442986731, 2.1844512147396244, 1.2000000000000006], [33.69042505267091, 80.06731529671714, 2.2022522716404778, 1.2000000000000006], [29.157427120978678, 82.5346645544511, 2.2146082993716583, 1.2000000000000006], [27.17382907061827, 93.78874887901951, 2.425079619199396, 1.2000000000000006], [34.761055666251615, 92.88790635480824, 2.4590063394104344, 1.2000000000000006], [-2.729118001525531, 22.918683596868465, 0.31309748555697403, -0.3999999999999999], [9.124522914489708, 21.80096170236561, 0.3072332269066863, -0.3999999999999999], [-1.5170192378515415, 28.303045293335575, 0.2765156815956554, -0.3999999999999999], [-1.3900091234452605, 30.022954081648294, 0.2645777264861412, -0.3999999999999999], [4.034616118215339, 61.19769858054814, 0.04620390436590388, -0.3999999999999999], [26.121526235859253, 82.71602090547535, 2.197226090868472, 1.2000000000000006]]
  in  "lane width":dbl=3.5
  out "XY Graph":cluster{"Y":dbl[], "Y":dbl[]}[](graph)
  out "seed_y":dbl[](array[numeric])
  out "seed_x":dbl[](array[numeric])
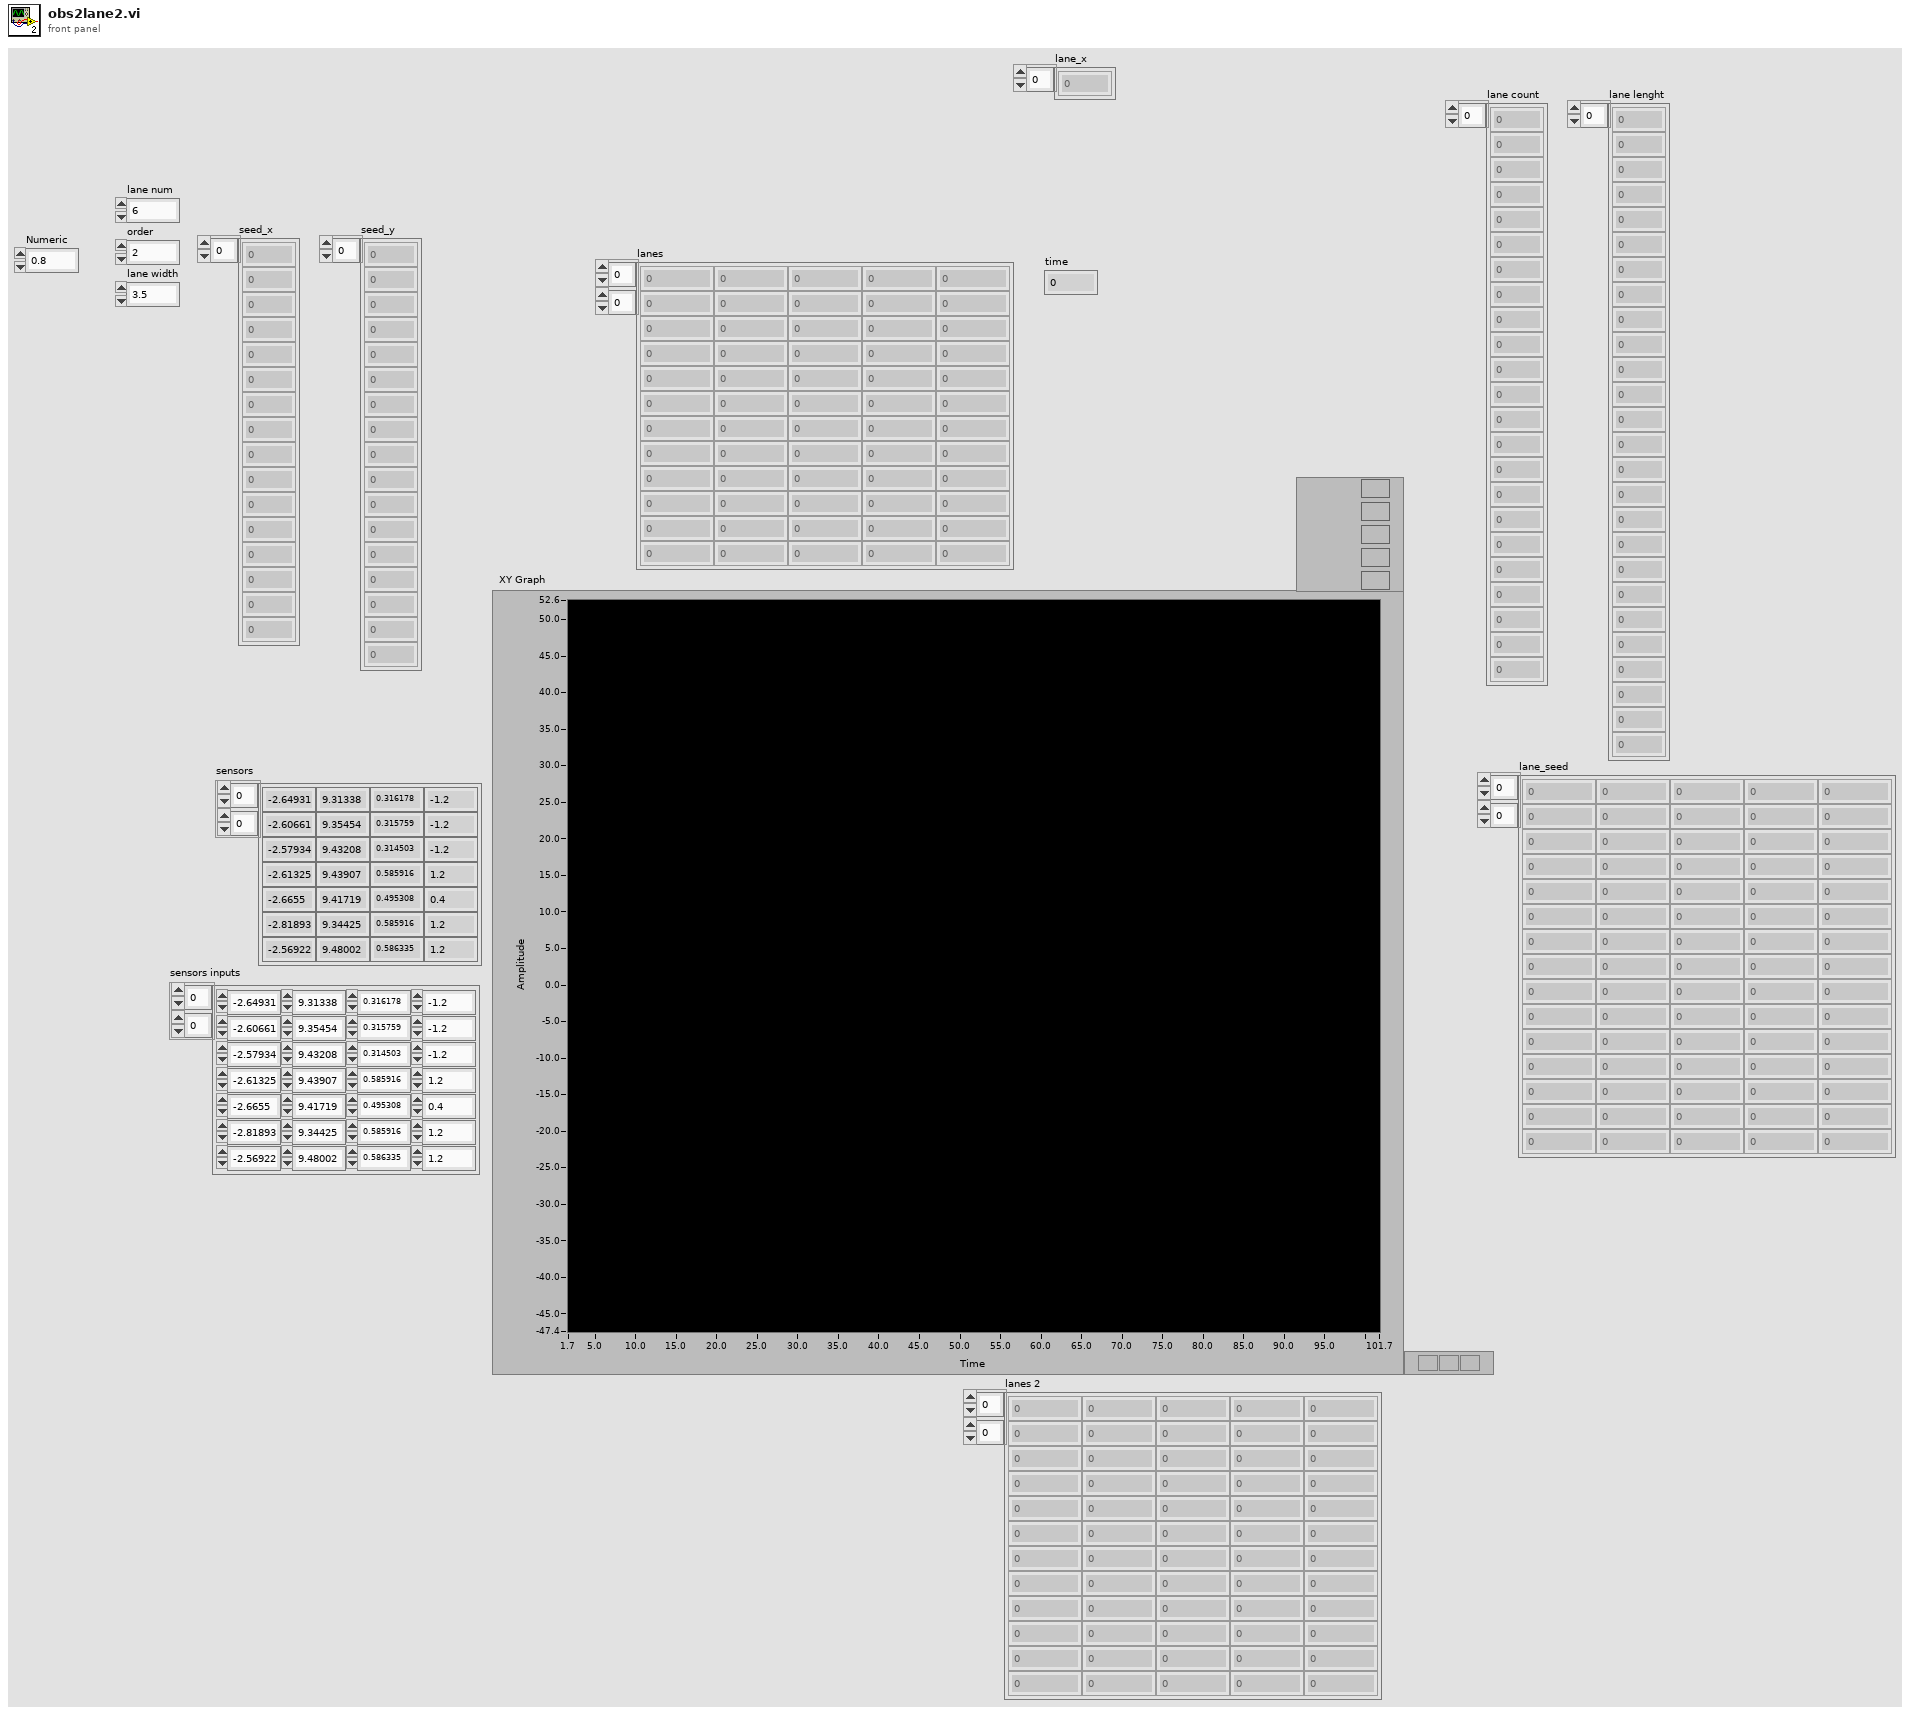
[diagram p1: front panel]
types:
  T1 = cluster{i16, "element":dbl, "element":dbl, "element":dbl}[]
  T2 = typedef "NI_Matrix.lvlib/RealMatrix.ctl" = dbl[][]
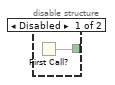
[diagram p3: hidden frame]
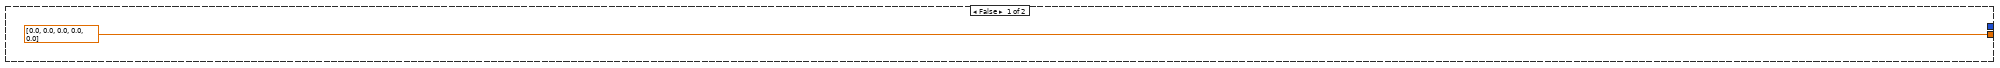
[diagram p5: hidden frame]
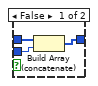
[diagram p7: hidden frame]
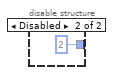
[diagram p9: hidden frame]
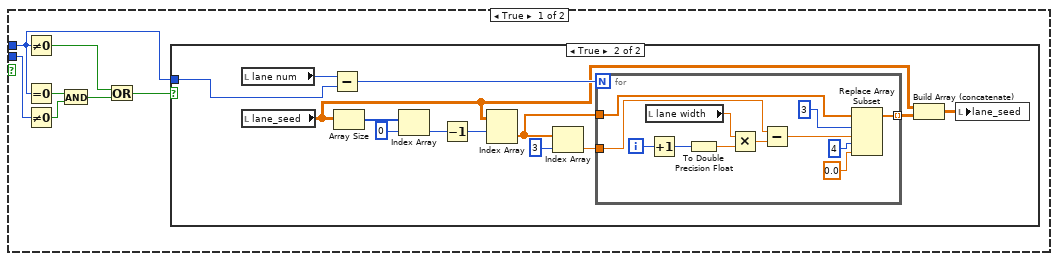
[diagram p14: hidden frame]
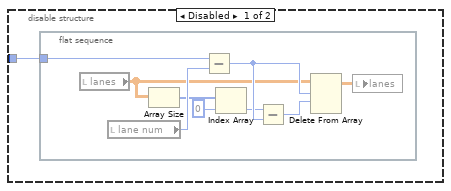
[diagram p16: hidden frame]
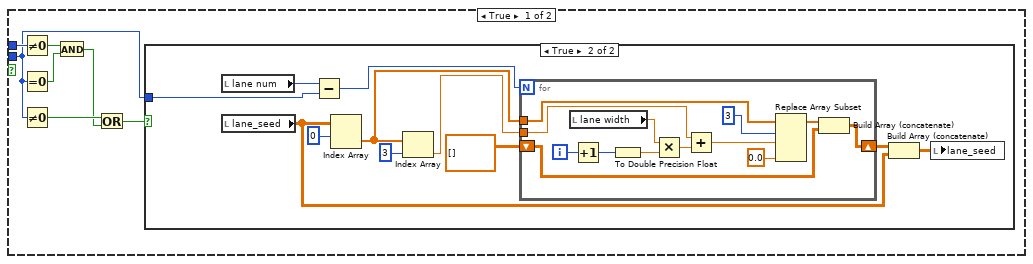
[diagram p17: hidden frame]
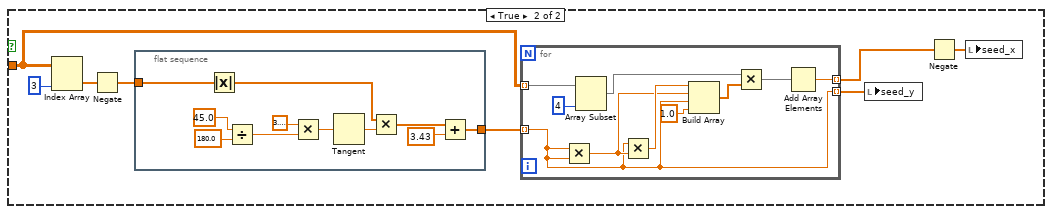
[diagram p20: hidden frame]
diagram:
  n1 = flat-sequence {
    tunnel: [w3] -> w2
    tunnel: w2 -> [w5]
    tunnel: [w5] -> w1
    tunnel: w1 -> [w840]
    frame #0 {
      n2 = Tick Count (ms)() -> (millisecond timer value=w3:u32)
    }
    frame #1 {
      n3 = flat-sequence {
        tunnel: [w126] -> w4
        tunnel: w4 -> [w143]
        frame #0 {
          n4 = disable-structure shown="Enabled" {
            disable-tunnel: [w19 _] -> w6
            frame Enabled {
              n5 = global read "G_SEN.vi" "sensor_lane"() -> (w14:dbl[][])
              n6 = global read "G_SEN.vi" "sensor_obs"() -> (w16:dbl[][])
              n7 = global read "G_SEN.vi" "sensor_velodyne_chopped"() -> (w18:dbl[][])
              n8 = flat-sequence {
                tunnel: w16 -> [w40]
                tunnel: [w27] -> w15
                frame #0 {
                  n9 = Index Array(array=w40, index (col) #1=2 ("disabled index (col)"), index (col) #2=0 ("index (col)")) -> (element #1=w38:dbl[], element #2=w34:dbl[], element #3=w33:dbl[], element #4=w21:dbl[])  [unwired: 6 in]
                  n10 = Greater?(x=w38, y=1.0) -> (0:w26:bool[])
                  n11 = Not(x=w26) -> (.not. x?=w25:bool[])
                  n12 = Boolean To (0,1)(Boolean=w26) -> (0, 1=w36:i16[])
                  n13 = Build Cluster Array(w36, w34, w33, w21) -> (w32:T1)
                  n14 = Boolean To (0,1)(Boolean=w25) -> (0, 1=w24:i16[])
                  n15 = To Long Integer(number=w24) -> (32bit integer=w23:i32[])
                  n16 = Sort 1D Array(array=w32) -> (sorted array=w31:T1)
                  n17 = Add Array Elements(numeric array=w23) -> (sum=w22:i32)
                  n18 = for {
                    N: w22 -> [_]
                    tunnel: w31 -> [w44] mode=indexing
                    tunnel: [w43] -> w30 mode=indexing
                    tunnel: [w42] -> w29 mode=indexing
                    tunnel: [w41] -> w20 mode=indexing
                    n19 = Unbundle(w44) -> ("element"=w43:dbl, "element"=w42:dbl, "element"=w41:dbl)  [unwired: 1 out]
                  }
                  n20 = Build Array(w30, w29, w20) -> (w28:dbl[][])
                  n21 = Transpose 2D Array(2D array=w28) -> (transposed array=w27:dbl[][])
                }
              }
              n22 = flat-sequence {
                tunnel: w18 -> [w65]
                tunnel: [w52] -> w17
                frame #0 {
                  n23 = Index Array(array=w65, index (col) #1=2 ("disabled index (col)"), index (col) #2=0 ("index (col)")) -> (element #1=w63:dbl[], element #2=w59:dbl[], element #3=w58:dbl[], element #4=w46:dbl[])  [unwired: 6 in]
                  n24 = Greater?(x=w63, y=2.0) -> (0:w48:bool[])
                  n25 = Not(x=w48) -> (.not. x?=w49:bool[])
                  n26 = Boolean To (0,1)(Boolean=w48) -> (0, 1=w61:i16[])
                  n27 = Boolean To (0,1)(Boolean=w49) -> (0, 1=w50:i16[])
                  n28 = Build Cluster Array(w61, w59, w58, w46) -> (w57:T1)
                  n29 = To Long Integer(number=w50) -> (32bit integer=w51:i32[])
                  n30 = Sort 1D Array(array=w57) -> (sorted array=w56:T1)
                  n31 = Add Array Elements(numeric array=w51) -> (sum=w47:i32)
                  n32 = for {
                    N: w47 -> [_]
                    tunnel: w56 -> [w69] mode=indexing
                    tunnel: [w68] -> w55 mode=indexing
                    tunnel: [w67] -> w54 mode=indexing
                    tunnel: [w66] -> w45 mode=indexing
                    n33 = Unbundle(w69) -> ("element"=w68:dbl, "element"=w67:dbl, "element"=w66:dbl)  [unwired: 1 out]
                  }
                  n34 = Build Array(w55, w54, w45) -> (w53:dbl[][])
                  n35 = Transpose 2D Array(2D array=w53) -> (transposed array=w52:dbl[][])
                }
              }
              n36 = Array Subset(array=w14, index (col)=0 ("index"), length (col)=3 ("length")) -> (w11:dbl[][])  [unwired: 2 in]
              n37 = Array Subset(array="sensors inputs", index (col)=0 ("index"), length (col)=3 ("length")) -> (w7:dbl[][])  [unwired: 2 in]
              n38 = Build Array (concatenate)(w15, w11, w17, w7) -> (w19:dbl[][])
            }
            frame Disabled {
            }
          }
          "sensors" <- w6
        }
        frame #1 {
          n39 = disable-structure shown="Enabled" {
            disable-tunnel: [w71 _] -> w70
            frame Disabled {
              n40 = First Call?() -> (First Call?: T/F=w71:bool)
            }
            frame Enabled {
            }
          }
          n41 = case shown="True" w70 {
            frame False {
            }
            frame True {
              n42 = local read "lane width"() -> (w77:dbl)
              n43 = local read "lane num"() -> (w73:i32)
              n44 = local write "lane width"(3.3 ("lane width")) -> ()
              n45 = for {
                N: 1000 -> [_]
                tunnel: [w96] -> w75 mode=indexing
                i -> [w99]
                n46 = To Double Precision Float(number=w99) -> (double precision float=w98:dbl)
                n47 = Multiply(x=0.1, y=w98) -> (x*y=w96:dbl)
              }
              "lane_x" <- w75
              n48 = Multiply(x=0.5, y=w77) -> (x*y=w83:dbl)
              n49 = for {
                N: w73 -> [_]
                tunnel: w77 -> [w105]
                tunnel: w83 -> [w101]
                tunnel: [w100] -> w80 mode=indexing
                i -> [w104]
                n50 = To Double Precision Float(number=w104) -> (double precision float=w103:dbl)
                n51 = Multiply(x=w105, y=w103) -> (x*y=w102:dbl)
                n52 = Add(x=w101, y=w102) -> (x+y=w100:dbl)
              }
              n53 = Reverse 1D Array(array=w80) -> (reversed array=w82:dbl[])
              n54 = Negate(x=w82) -> (-x=w81:dbl[])
              n55 = Build Array (concatenate)(w81, w80) -> (w78:dbl[])
              n56 = flat-sequence {
                tunnel: [w87] -> w79
                tunnel: w78 -> [w85]
                tunnel: [w85] -> w74
                frame #0 {
                  n57 = Divide(x=45.0, y=180.0) -> (x/y=w92:dbl)
                  n58 = Multiply(x=3.141592653589793, y=w92) -> (x*y=w91:dbl)
                  n59 = Absolute Value(x=w85) -> (abs(x)=w86:dbl[])
                  n60 = Tangent(1:w91) -> (0:w90:dbl)
                  n61 = Multiply(x=w86, y=w90) -> (x*y=w89:dbl[])
                  n62 = Add(x=w89, y=3.43) -> (x+y=w87:dbl[])
                }
              }
              "seed_x" <- w74
              "seed_y" <- w79
            }
          }
        }
        frame #2 {
          n63 = local read "lane width"() -> (w119:dbl)
          n64 = local read "sensors"() -> (w107:dbl[][])
          n65 = local read "sensors"() -> (w106:dbl[][])
          n66 = Index Array(array=w107, index (col)=0 ("disabled index (col)")) -> (element=w124:dbl[])  [unwired: 1 in]
          n67 = Index Array(array=w106, index (col)=1 ("disabled index (col)")) -> (element=w122:dbl[])  [unwired: 1 in]
          n68 = local read "seed_x"() -> (w128:dbl[])
          n69 = local read "seed_y"() -> (w127:dbl[])
          n70 = for {
            tunnel: w128 -> [w140] mode=indexing
            tunnel: w124 -> [w141]
            tunnel: [w138] -> w116 mode=indexing
            tunnel: w127 -> [w137] mode=indexing
            tunnel: w122 -> [w136]
            tunnel: [w135] -> w121 mode=indexing
            n71 = Subtract(x=w141, y=w140) -> (x-y=w139:dbl[])
            n72 = Subtract(x=w137, y=w136) -> (x-y=w131:dbl[])
            n73 = Multiply(x=w131, y=0.25) -> (x*y=w129:dbl[])
            n74 = Square(x=w139) -> (x^2=w134:dbl[])
            n75 = Square(x=w129) -> (x^2=w132:dbl[])
            n76 = Add(x=w134, y=w132) -> (x+y=w133:dbl[])
            n77 = Array Max & Min(array=w133) -> (min value=w135:dbl, min index (indices)=w138:i32)  [unwired: 2 out]
          }
          n78 = Square Root(x=w121) -> (sqrt(x)=w108:dbl[])
          n79 = Multiply(x=0.8, y=w119) -> (x*y=w109:dbl)
          n80 = Greater?(x=w109, y=w108) -> (0:w115:bool[])
          n81 = Not(x=w115) -> (.not. x?=w114:bool[])
          n82 = Boolean To (0,1)(Boolean=w115) -> (0, 1=w118:i16[])
          n83 = Boolean To (0,1)(Boolean=w114) -> (0, 1=w113:i16[])
          n84 = To Long Integer(number=w118) -> (32bit integer=w117:i32[])
          n85 = To Long Integer(number=w113) -> (32bit integer=w112:i32[])
          n86 = Multiply(x=w117, y=w116) -> (x*y=w110:i32[])
          n87 = Negate(x=w112) -> (-x=w111:i32[])
          n88 = Add(x=w111, y=w110) -> (x+y=w126:i32[])
        }
        frame #3 {
          n89 = local read "lane width"() -> (w149:dbl)
          n90 = local read "sensors"() -> (w147:dbl[][])
          n91 = Index Array(array=w147, index (col)=1 ("disabled index (col)")) -> (element=w152:dbl[])  [unwired: 1 in]
          n92 = Multiply(x=w149, y=0.01) -> (x*y=w151:dbl)
          n93 = Multiply(x=w151, y=w152) -> (x*y=w154:dbl[])
          n94 = Max & Min(x=0.3 ("y"), y=w154) -> (max(x,y)=w146:dbl[])  [unwired: 1 out]
          n95 = for {
            tunnel: w143 -> [w160] mode=indexing
            tunnel: w146 -> [w159]
            tunnel: [w158] -> w145 mode=indexing
            tunnel: [w157] -> w144 mode=indexing
            tunnel: [w155] -> w142 mode=indexing
            i -> [w156]
            n96 = Greater Or Equal To 0?(x=w160) -> (x >= 0?=w161:bool)
            n97 = case shown="True" w161 {
              tunnel: w160 -> [_ w181]
              tunnel: w159 -> [_ w182]
              tunnel: [dbl[] [0.0, 0.0, 0.0, 0.0, 0.0] w166] -> w158
              tunnel: [_ w165] -> w157
              tunnel: w156 -> [_ _]
              tunnel: [_ w163] -> w155
              frame False {
              }
              frame True {
                n98 = local read "sensors"() -> (w180:dbl[][])
                n99 = Index Array(array=w180, index (col) #1=1 ("disabled index (col)"), index (col) #2=0 ("disabled index (col)")) -> (element #1=w172:dbl[], element #2=w177:dbl[])  [unwired: 2 in]
                n100 = Index Array(array=w177, index=w181) -> (element=w175:dbl)
                n101 = Subtract(x=w177, y=w175) -> (x-y=w178:dbl[])
                n102 = Absolute Value(x=w178) -> (abs(x)=w176:dbl[])
                n103 = Less?(x=w176, y=w182) -> (x < y?=w170:bool[])
                n104 = Greater?(x=100.0 ("y"), y=w172) -> (0:w171:bool[])
                n105 = And(x=w171, y=w170) -> (x .and. y?=w169:bool[])
                n106 = for {
                  N: 3 -> [_]
                  tunnel: [w194] -> w167
                  shift-right: [w192] -> _
                  shift-left: w169 -> [w193]
                  tunnel: [w191] -> w165
                  tunnel: [w190] -> w164
                  tunnel: [w189] -> w163
                  stop <- w190 stop-if-true
                  n107 = flat-sequence {
                    tunnel: [w221] -> w194
                    tunnel: w193 -> [w226]
                    tunnel: [w227] -> w192
                    frame #0 {
                      n108 = local read "order"() -> (w217:i32)
                      n109 = Boolean To (0,1)(Boolean=w226) -> (0, 1=w244:i16[])
                      n110 = local read "sensors"() -> (w231:dbl[][])
                      n111 = local read "sensors"() -> (w240:dbl[][])
                      n112 = Array Subset(array=dbl[] [0.0, 0.0], index=0, length=w217) -> (w215:dbl[])
                      n113 = To Double Precision Float(number=w244) -> (double precision float=w237:dbl[])
                      n114 = Index Array(array=w231, index (col)=1 ("disabled index (col)")) -> (element=w230:dbl[])  [unwired: 1 in]
                      n115 = Index Array(array=w240, index (col)=0 ("disabled index (col)")) -> (element=w236:dbl[])  [unwired: 1 in]
                      n116 = Multiply(x=w230, y=w237) -> (x*y=w234:dbl[])
                      n117 = Negate(x=w236) -> (-x=w233:dbl[])
                      n118 = Multiply(x=w237, y=w233) -> (x*y=w235:dbl[])
                      n119 = flat-sequence {
                        tunnel: [w294] -> w243
                        tunnel: w237 -> [w293]
                        tunnel: w234 -> [w292]
                        frame #0 {
                          n120 = Multiply(x=w292, y=w292) -> (x*y=w284:dbl[])
                          n121 = Add Array Elements(numeric array=w293) -> (sum=w280:dbl)
                          n122 = Multiply(x=w292, y=w284) -> (x*y=w288:dbl[])
                          n123 = Add Array Elements(numeric array=w284) -> (sum=w290:dbl)
                          n124 = Multiply(x=w292, y=w288) -> (x*y=w286:dbl[])
                          n125 = Add Array Elements(numeric array=w288) -> (sum=w289:dbl)
                          n126 = Multiply(x=w292, y=w286) -> (x*y=w282:dbl[])
                          n127 = Add Array Elements(numeric array=w286) -> (sum=w287:dbl)
                          n128 = Multiply(x=w292, y=w282) -> (x*y=w283:dbl[])
                          n129 = Add Array Elements(numeric array=w282) -> (sum=w285:dbl)
                          n130 = Add Array Elements(numeric array=w283) -> (sum=w281:dbl)
                          n131 = Add Array Elements(numeric array=w292) -> (sum=w291:dbl)
                          n132 = Build Array(w281, w285, w287, w289, w290, w291, w280) -> (w294:dbl[])
                        }
                      }
                      n133 = flat-sequence {
                        tunnel: w234 -> [w279]
                        tunnel: w235 -> [w277]
                        tunnel: [w270] -> w223
                        frame #0 {
                          n134 = Multiply(x=w279, y=w277) -> (x*y=w275:dbl[])
                          n135 = Add Array Elements(numeric array=w277) -> (sum=w278:dbl)
                          n136 = Multiply(x=w279, y=w275) -> (x*y=w272:dbl[])
                          n137 = Add Array Elements(numeric array=w275) -> (sum=w276:dbl)
                          n138 = Multiply(x=w279, y=w272) -> (x*y=w273:dbl[])
                          n139 = Add Array Elements(numeric array=w272) -> (sum=w274:dbl)
                          n140 = Add Array Elements(numeric array=w273) -> (sum=w271:dbl)
                          n141 = Build Array(w271, w274, w276, w278) -> (w270:dbl[])
                        }
                      }
                      n142 = local read "order"() -> (w220:i32)
                      n143 = for {
                        N: 4 -> [_]
                        tunnel: w243 -> [w298]
                        tunnel: [w295] -> w225 mode=indexing
                        i -> [w297]
                        n144 = Array Subset(array=w298, index=w297, length=4) -> (w295:dbl[])
                      }
                      n145 = local read "order"() -> (w219:i32)
                      n146 = Array Subset(array=w225, index (row)=w219, index (col)=w219) -> (w224:dbl[][])  [unwired: 2 in]
                      n147 = call-poly <vilib>:"Array To Matrix.vi"("Real 2D Array"=w224) -> ("Real Matrix"=w239:T2)
                      n148 = call-poly <vilib>:"Inverse Matrix.vi"("Input Matrix"=w239) -> ("Inverse Matrix"=w238:T2)  [unwired: 1 in, 1 out]
                      n149 = Array Subset(array=w223, index=w220) -> (w222:dbl[])  [unwired: 1 in]
                      n150 = call-poly <vilib>:"A x B.vi"("Vector"=w222, "A"=w238) -> ("A x Vector"=w229:dbl[])  [unwired: 1 out]
                      n151 = Build Array (concatenate)(w215, w229, 1.0) -> (w221:dbl[])
                      n152 = flat-sequence {
                        tunnel: w221 -> [w259]
                        tunnel: [w247] -> w227
                        tunnel: w226 -> [w246]
                        frame #0 {
                          n153 = local read "sensors"() -> (w253:dbl[][])
                          n154 = local read "sensors"() -> (w250:dbl[][])
                          n155 = Index Array(array=w259, index #1=0 ("index")) -> (element #1=w263:dbl, element #2=w264:dbl, element #3=w265:dbl, element #4=w269:dbl)  [unwired: 3 in]
                          n156 = Index Array(array=w253, index (col)=1 ("disabled index (col)")) -> (element=w252:dbl[])  [unwired: 1 in]
                          n157 = Index Array(array=w250, index (col)=0 ("disabled index (col)")) -> (element=w251:dbl[])  [unwired: 1 in]
                          n158 = Multiply(x=w252, y=w265) -> (x*y=w268:dbl[])
                          n159 = Multiply(x=w252, y=w252) -> (x*y=w261:dbl[])
                          n160 = Negate(x=w251) -> (-x=w248:dbl[])
                          n161 = Multiply(x=w261, y=w264) -> (x*y=w267:dbl[])
                          n162 = Multiply(x=w252, y=w261) -> (x*y=w262:dbl[])
                          n163 = Multiply(x=w262, y=w263) -> (x*y=w266:dbl[])
                          n164 = Compound Arithmetic op=ADD(w266, w267, w268, w269) -> (w258:dbl[])
                          n165 = Subtract(x=w258, y=w248) -> (x-y=w257:dbl[])
                          n166 = Absolute Value(x=w257) -> (abs(x)=w256:dbl[])
                          n167 = Less?(x=w256, y=0.5) -> (x < y?=w245:bool[])
                          n168 = And(x=w246, y=w245) -> (x .and. y?=w247:bool[])
                        }
                      }
                    }
                  }
                  n169 = flat-sequence {
                    tunnel: w192 -> [w209]
                    tunnel: [w213] -> w191
                    tunnel: [w196] -> w190
                    tunnel: [w195] -> w189
                    frame #0 {
                      n170 = Boolean To (0,1)(Boolean=w209) -> (0, 1=w210:i16[])
                      n171 = Not(x=w209) -> (.not. x?=w208:bool[])
                      n172 = local read "sensors"() -> (w212:dbl[][])
                      n173 = Add Array Elements(numeric array=w210) -> (sum=w213:i16)
                      n174 = Boolean To (0,1)(Boolean=w208) -> (0, 1=w207:i16[])
                      n175 = Index Array(array=w212, index (col)=1 ("disabled index (col)")) -> (element=w206:dbl[])  [unwired: 1 in]
                      n176 = Multiply(x=w206, y=w210) -> (x*y=w203:dbl[])
                      n177 = Multiply(x=999.0, y=w207) -> (x*y=w204:dbl[])
                      n178 = Add(x=w203, y=w204) -> (x+y=w202:dbl[])
                      n179 = Array Max & Min(array=w203) -> (max value=w200:dbl)  [unwired: 3 out]
                      n180 = Array Max & Min(array=w202) -> (min value=w201:dbl)  [unwired: 3 out]
                      n181 = Subtract(x=w200, y=w201) -> (x-y=w195:dbl)
                      n182 = Less?(x=w213, y=i16 70) -> (x < y?=w198:bool)
                      n183 = Less?(x=w195, y=14.0) -> (x < y?=w197:bool)
                      n184 = Or(x=w198, y=w197) -> (x .or. y?=w196:bool)
                    }
                  }
                }
                n185 = flat-sequence {
                  tunnel: w167 -> [w186]
                  tunnel: [w188] -> w166
                  tunnel: w164 -> [w187]
                  frame #0 {
                    n186 = Replace Array Subset(array=w186, new element=0.0 ("new element/subarray"), index=4) -> (w184:dbl[])
                    n187 = Select(t=w184, s=w187, f=w186) -> (s? t:f=w188:dbl[])
                  }
                }
              }
            }
          }
          "lanes" <- w145
          "lane count" <- w144
          "lane lenght" <- w142
        }
        frame #4 {
          n188 = local read "lanes"() -> (w304:dbl[][])
          n189 = Index Array(array=w304, index (col)=4 ("disabled index (col)")) -> (element=w301:dbl[])  [unwired: 1 in]
          n190 = Array Size(array=w301) -> (size(s)=w300:i32)
          n191 = for {
            N: w300 -> [_]
            shift-right: [w310] -> w299
            shift-left: dbl[][] [] -> [w309]
            shift-right: [w305] -> _
            shift-left: w301 -> [w306]
            i -> [w308]
            n192 = Index Array(array=w306, index=w308) -> (element=w307:dbl)
            n193 = Not Equal To 0?(x=w307) -> (x != 0?=w311:bool)
            n194 = case shown="True" w311 {
              tunnel: w308 -> [_ w329]
              tunnel: [w313 w328] -> w310
              tunnel: w309 -> [w313 w327]
              tunnel: w306 -> [w312 w325]
              tunnel: [w312 w324] -> w305
              frame False {
              }
              frame True {
                n195 = local read "lanes"() -> (w323:dbl[][])
                n196 = Index Array(array=w323, index (col)=3 ("disabled index (col)")) -> (element=w314:dbl[])  [unwired: 1 in]
                n197 = Index Array(array=w314, index=w329) -> (element=w315:dbl)
                n198 = Equal?(x=w315, y=w314) -> (x = y?=w321:bool[])
                n199 = Boolean To (0,1)(Boolean=w321) -> (0, 1=w326:i16[])
                n200 = To Double Precision Float(number=w326) -> (double precision float=w317:dbl[])
                n201 = Array Max & Min(array=w326) -> (max index (indices)=w319:i32)  [unwired: 3 out]
                n202 = local read "lanes"() -> (w320:dbl[][])
                n203 = Subtract(x=w325, y=w317) -> (x-y=w316:dbl[])
                n204 = Replace Array Subset(array=w325, new element=w316) -> (w324:dbl[])  [unwired: 1 in]
                n205 = Index Array(array=w320, index (row)=w319) -> (element=w318:dbl[])  [unwired: 1 in]
                n206 = Build Array (concatenate)(w327, w318) -> (w328:dbl[][])
              }
            }
          }
          n207 = local write "lanes"(w299) -> ()
        }
        frame #5 {
          n208 = Build Array(1000000.0 ("element"), 10000.0 ("element"), 100.0 ("element"), 1.0 ("element")) -> (w339:dbl[])
          n209 = local read "lanes"() -> (w340:dbl[][])
          n210 = for {
            tunnel: w340 -> [w359] mode=indexing
            tunnel: w339 -> [w362]
            tunnel: [w360] -> w338 mode=indexing
            tunnel: [w358] -> w337 mode=indexing
            i -> [w358]
            n211 = Array Subset(array=w359, index=0, length=4) -> (w363:dbl[])
            n212 = Multiply(x=w362, y=w363) -> (x*y=w361:dbl[])
            n213 = Add Array Elements(numeric array=w361) -> (sum=w360:dbl)
          }
          n214 = Build Cluster Array(w338, w337) -> (w336:cluster{dbl, i32}[])
          n215 = Sort 1D Array(array=w336) -> (sorted array=w335:cluster{dbl, i32}[])
          n216 = Reverse 1D Array(array=w335) -> (reversed array=w334:cluster{dbl, i32}[])
          n217 = for {
            tunnel: w334 -> [w353] mode=indexing
            shift-right: [w349] -> w332
            shift-left: i32[] [] -> [w348]
            i -> [w352]
            n218 = Unbundle(w353) -> (w350:i32)  [unwired: 1 out]
            n219 = Greater?(x=w350, y=w352) -> (0:w351:bool)
            n220 = case shown="True" w351 {
              tunnel: w350 -> [w356 _]
              tunnel: [w355 w357] -> w349
              tunnel: w348 -> [w354 w357]
              frame False {
                n221 = Build Array (concatenate)(w354, w356) -> (w355:i32[])
              }
              frame True {
              }
            }
          }
          n222 = local read "lanes"() -> (w331:dbl[][])
          n223 = for {
            tunnel: w332 -> [w346] mode=indexing
            tunnel: w331 -> [w347]
            tunnel: [w345] -> w330 mode=indexing
            n224 = Index Array(array=w347, index (row)=w346) -> (element=w345:dbl[])  [unwired: 1 in]
          }
          n225 = local write "lanes"(w330) -> ()
        }
        frame #6 {
          n226 = local read "lanes"() -> (w384:dbl[][])
          n227 = local read "lane width"() -> (w375:dbl)
          n228 = Index Array(array=w384, index (col)=3 ("disabled index (col)")) -> (element=w379:dbl[])  [unwired: 1 in]
          n229 = Array Size(array=w379) -> (size(s)=w381:i32)
          n230 = Decrement(x=w381) -> (x-1=w380:i32)
          n231 = Array Subset(array=w379, index=1) -> (w376:dbl[])  [unwired: 1 in]
          n232 = Array Subset(array=w379, index=0, length=w380) -> (w377:dbl[])
          n233 = Subtract(x=w377, y=w376) -> (x-y=w372:dbl[])
          n234 = Subtract(x=w372, y=w375) -> (x-y=w374:dbl[])
          n235 = Absolute Value(x=w374) -> (abs(x)=w373:dbl[])
          n236 = Array Max & Min(array=w373) -> (min index (indices)=w371:i32)  [unwired: 3 out]
          n237 = Index Array(array=w372, index=w371) -> (element=w366:dbl)
          n238 = In Range and Coerce(upper limit=4.2, x=w366, lower limit=2.8) -> (coerced(x)=w370:dbl, In Range?=w369:bool)
          n239 = case shown="True" w369 {
            tunnel: w370 -> [_ w389]
            frame False {
            }
            frame True {
              n240 = local read "lane width"() -> (w388:dbl)
              n241 = Add(x=w389, y=w388) -> (x+y=w387:dbl)
              n242 = Multiply(x=w387, y=0.5) -> (x*y=w385:dbl)
              n243 = local write "lane width"(w385) -> ()
            }
          }
        }
        frame #7 {
          n244 = local read "lanes"() -> (w390:dbl[][])
          "lanes 2" <- w390
          n245 = Array Subset(array=w390, index (row)=0 ("index"), length (row)=1 ("length")) -> (w394:dbl[][])  [unwired: 2 in]
          n246 = Array Subset(array=w390, index (row)=1 ("index")) -> (w393:dbl[][])  [unwired: 3 in]
          n247 = disable-structure shown="Enabled" {
            disable-tunnel: w393 -> [w399 _]
            disable-tunnel: [w398 2] -> w391
            frame Enabled {
              n248 = Array Size(array=w399) -> (size(s)=w401:i32[])
              n249 = Index Array(array=w401, index=0) -> (element=w398:i32)
            }
            frame Disabled {
            }
          }
          n250 = for {
            N: w391 -> [_]
            shift-right: [w409] -> w392
            shift-left: w394 -> [w412]
            tunnel: w393 -> [w410] mode=indexing
            n251 = Array Size(array=w412) -> (size(s)=w421:i32[])
            n252 = Index Array(array=w410, index=3) -> (element=w415:dbl)
            n253 = local read "lane width"() -> (w414:dbl)
            n254 = Index Array(array=w421, index=0) -> (element=w420:i32)
            n255 = Decrement(x=w420) -> (x-1=w419:i32)
            n256 = Index Array(array=w412, index (row)=w419, index (col)=3 ("disabled index (col)")) -> (element=w416:dbl)
            n257 = Subtract(x=w416, y=w415) -> (x-y=w407:dbl)
            n258 = Divide(x=w407, y=w414) -> (x/y=w413:dbl)
            n259 = Round To Nearest(number=w413) -> (nearest integer value=w408:dbl)
            n260 = Divide(x=w407, y=w408) -> (x/y=w406:dbl)
            n261 = In Range and Coerce(upper limit=4.2, x=w406, lower limit=2.8) -> (In Range?=w403:bool)  [unwired: 1 out]
            n262 = case shown="True" w403 {
              tunnel: w412 -> [w423 w426]
              tunnel: [w423 w425] -> w411
              tunnel: w408 -> [_ w424]
              frame False {
              }
              frame True {
                n263 = Decrement(x=w424) -> (x-1=w427:dbl)
                n264 = for {
                  N: w427 -> [_]
                  shift-right: [w429] -> w425
                  shift-left: w426 -> [w430]
                  n265 = Build Array (concatenate)(w430, dbl[] [0.0, 0.0, 0.0, 0.0, 0.0]) -> (w429:dbl[][])
                }
              }
            }
            n266 = Build Array (concatenate)(w411, w410) -> (w409:dbl[][])
          }
          n267 = local write "lanes"(w392) -> ()
        }
        frame #8 {
          n268 = local read "lanes"() -> (w433:dbl[][])
          n269 = Index Array(array=w433, index (col)=4 ("disabled index (col)")) -> (element=w431:dbl[])  [unwired: 1 in]
          n270 = for {
            tunnel: w431 -> [w437] mode=indexing
            tunnel: w431 -> [w434]
            i -> [w435]
            n271 = Equal To 0?(x=w437) -> (x = 0?=w436:bool)
            n272 = case shown="True" w436 {
              tunnel: w435 -> [_ w439]
              tunnel: w434 -> [_ w438]
              frame False {
              }
              frame True {
                n273 = Increment(x=w439) -> (x+1=w445:i32)
                n274 = Array Subset(array=w438, index=w445) -> (w453:dbl[])  [unwired: 1 in]
                n275 = Array Subset(array=w438, index=0, length=w439) -> (w451:dbl[])
                n276 = Array Max & Min(array=w453) -> (max value=w452:dbl, max index (indices)=w446:i32)  [unwired: 2 out]
                n277 = Reverse 1D Array(array=w451) -> (reversed array=w444:dbl[])
                n278 = Array Max & Min(array=w444) -> (max value=w450:dbl, max index (indices)=w442:i32)  [unwired: 2 out]
                n279 = Array Size(array=w444) -> (size(s)=w443:i32)
                n280 = Not Equal To 0?(x=w452) -> (x != 0?=w448:bool)
                n281 = Not Equal To 0?(x=w450) -> (x != 0?=w449:bool)
                n282 = Subtract(x=w443, y=w442) -> (x-y=w441:i32)
                n283 = Decrement(x=w441) -> (x-1=w440:i32)
                n284 = And(x=w449, y=w448) -> (x .and. y?=w447:bool)
                n285 = case shown="True" w447 {
                  tunnel: w446 -> [_ w474]
                  tunnel: w445 -> [_ w473]
                  tunnel: w440 -> [_ w472]
                  tunnel: w439 -> [_ w471]
                  frame False {
                  }
                  frame True {
                    n286 = local read "lanes"() -> (w457:dbl[][])
                    n287 = Subtract(x=w472, y=w471) -> (x-y=w470:i32)
                    n288 = Add(x=w474, y=w473) -> (x+y=w465:i32)
                    n289 = Subtract(x=w471, y=w465) -> (x-y=w469:i32)
                    n290 = Subtract(x=w472, y=w465) -> (x-y=w468:i32)
                    n291 = Index Array(array=w457, index (row) #1=w472, index (row) #2=w465) -> (element #1=w467:dbl[], element #2=w464:dbl[])  [unwired: 2 in]
                    n292 = Divide(x=w469, y=w468) -> (x/y=w466:dbl)
                    n293 = Divide(x=w470, y=w468) -> (x/y=w463:dbl)
                    n294 = Multiply(x=w467, y=w466) -> (x*y=w462:dbl[])
                    n295 = Multiply(x=w464, y=w463) -> (x*y=w461:dbl[])
                    n296 = Add(x=w462, y=w461) -> (x+y=w460:dbl[])
                    n297 = Replace Array Subset(array=w460, new element=0.0 ("new element/subarray"), index=4) -> (w455:dbl[])
                    n298 = Replace Array Subset(array=w457, new element=w455, index (row)=w471) -> (w456:dbl[][])  [unwired: 1 in]
                    n299 = local write "lanes"(w456) -> ()
                  }
                }
              }
            }
          }
        }
        frame #9 {
          n300 = local read "lanes"() -> (→"lane_seed":dbl[][])
        }
        frame #10 {
          n301 = for {
            N: 2 -> [_]
            n302 = flat-sequence {
              tunnel: [w483] -> w480
              tunnel: [w482] -> w479
              tunnel: w480 -> [w496]
              tunnel: [w498] -> w478
              tunnel: w479 -> [w498]
              tunnel: [w496] -> w477
              tunnel: w478 -> [w552]
              tunnel: w477 -> [w554]
              frame #0 {
                n303 = local read "lane_seed"() -> (w481:dbl[][])
                n304 = Index Array(array=w481, index (col)=3 ("disabled index (col)")) -> (element=w487:dbl[])  [unwired: 1 in]
                n305 = Array Size(array=w487) -> (size(s)=w486:i32)
                n306 = Greater?(x=w486, y=1) -> (0:w484:bool)
                n307 = case shown="True" w484 {
                  tunnel: w487 -> [_ w491]
                  tunnel: [_ w490] -> w483
                  tunnel: [_ w489] -> w482
                  frame False {
                  }
                  frame True {
                    n308 = Less Than 0?(x=w491) -> (x < 0?=w494:bool[])
                    n309 = Boolean To (0,1)(Boolean=w494) -> (0, 1=w493:i16[])
                    n310 = Array Size(array=w493) -> (size(s)=w492:i32)
                    n311 = Array Max & Min(array=w493) -> (max index (indices)=w489:i32)  [unwired: 3 out]
                    n312 = Subtract(x=w492, y=w489) -> (x-y=w490:i32)
                  }
                }
              }
              frame #1 {
                n313 = local read "lane num"() -> (w495:i32)
                n314 = Less Or Equal?(x=w496, y=w495) -> (x <= y?=w497:bool)
                n315 = case shown="False" w497 {
                  tunnel: w498 -> [w505 _]
                  tunnel: w496 -> [w499 w531]
                  frame True {
                    n316 = Not Equal To 0?(x=w499) -> (x != 0?=w501:bool)
                    n317 = Equal To 0?(x=w499) -> (x = 0?=w504:bool)
                    n318 = Not Equal To 0?(x=w505) -> (x != 0?=w503:bool)
                    n319 = And(x=w504, y=w503) -> (x .and. y?=w502:bool)
                    n320 = Or(x=w501, y=w502) -> (x .or. y?=w500:bool)
                    n321 = case shown="True" w500 {
                      tunnel: w499 -> [_ w507]
                      frame False {
                      }
                      frame True {
                        n322 = local read "lane num"() -> (w506:i32)
                        n323 = local read "lane_seed"() -> (w510:dbl[][])
                        n324 = Subtract(x=w506, y=w507) -> (x-y=w516:i32)
                        n325 = Array Size(array=w510) -> (size(s)=w518:i32[])
                        n326 = Index Array(array=w518, index=0) -> (element=w509:i32)
                        n327 = Decrement(x=w509) -> (x-1=w508:i32)
                        n328 = Index Array(array=w510, index (row)=w508) -> (element=w515:dbl[])  [unwired: 1 in]
                        n329 = Index Array(array=w515, index=3) -> (element=w513:dbl)
                        n330 = for {
                          N: w516 -> [_]
                          tunnel: w515 -> [w530]
                          tunnel: w513 -> [w524]
                          tunnel: [w521] -> w511 mode=indexing
                          i -> [w529]
                          n331 = local read "lane width"() -> (w527:dbl)
                          n332 = Increment(x=w529) -> (x+1=w528:i32)
                          n333 = To Double Precision Float(number=w528) -> (double precision float=w526:dbl)
                          n334 = Multiply(x=w527, y=w526) -> (x*y=w525:dbl)
                          n335 = Subtract(x=w524, y=w525) -> (x-y=w523:dbl)
                          n336 = Replace Array Subset(array=w530, new element #1=w523, index #1=3 ("index"), new element #2=0.0 ("new element/subarray"), index #2=4 ("index")) -> (w521:dbl[])
                        }
                        n337 = Build Array (concatenate)(w510, w511) -> (w512:dbl[][])
                        n338 = local write "lane_seed"(w512) -> ()
                      }
                    }
                  }
                  frame False {
                    n339 = disable-structure shown="Enabled" {
                      disable-tunnel: w531 -> [w532 _]
                      frame Disabled {
                        n340 = flat-sequence {
                          tunnel: w532 -> [w534]
                          frame #0 {
                            n341 = local read "lanes"() -> (w535:dbl[][])
                            n342 = local read "lane num"() -> (w541:i32)
                            n343 = Array Size(array=w535) -> (size(s)=w536:i32[])
                            n344 = Subtract(x=w534, y=w541) -> (x-y=w538:i32)
                            n345 = Index Array(array=w536, index=0) -> (element=w533:i32)
                            n346 = Subtract(x=w533, y=w538) -> (x-y=w539:i32)
                            n347 = Delete From Array(array=w535, length=w538, index (row)=w539) -> (array with subset deleted=w540:dbl[][])  [unwired: 1 in, 1 out]
                            n348 = local write "lanes"(w540) -> ()
                          }
                        }
                      }
                      frame Enabled {
                      }
                    }
                    n349 = flat-sequence {
                      tunnel: w531 -> [w543]
                      frame #0 {
                        n350 = local read "lane num"() -> (w544:i32)
                        n351 = local read "lane_seed"() -> (w550:dbl[][])
                        n352 = Subtract(x=w543, y=w544) -> (x-y=w547:i32)
                        n353 = Array Size(array=w550) -> (size(s)=w549:i32[])
                        n354 = Index Array(array=w549, index=0) -> (element=w542:i32)
                        n355 = Subtract(x=w542, y=w547) -> (x-y=w546:i32)
                        n356 = Delete From Array(array=w550, length=w547, index (row)=w546) -> (array with subset deleted=w545:dbl[][])  [unwired: 1 in, 1 out]
                        n357 = local write "lane_seed"(w545) -> ()
                      }
                    }
                  }
                }
              }
              frame #2 {
                n358 = local read "lane num"() -> (w553:i32)
                n359 = Less Or Equal?(x=w552, y=w553) -> (x <= y?=w551:bool)
                n360 = case shown="False" w551 {
                  tunnel: w554 -> [w561 _]
                  tunnel: w552 -> [w555 w586]
                  frame True {
                    n361 = Not Equal To 0?(x=w561) -> (x != 0?=w560:bool)
                    n362 = Equal To 0?(x=w555) -> (x = 0?=w559:bool)
                    n363 = Not Equal To 0?(x=w555) -> (x != 0?=w557:bool)
                    n364 = And(x=w560, y=w559) -> (x .and. y?=w556:bool)
                    n365 = Or(x=w557, y=w556) -> (x .or. y?=w558:bool)
                    n366 = case shown="True" w558 {
                      tunnel: w555 -> [_ w566]
                      frame False {
                      }
                      frame True {
                        n367 = local read "lane num"() -> (w562:i32)
                        n368 = local read "lane_seed"() -> (w572:dbl[][])
                        n369 = Subtract(x=w562, y=w566) -> (x-y=w567:i32)
                        n370 = Index Array(array=w572, index (row)=0) -> (element=w568:dbl[])  [unwired: 1 in]
                        n371 = Index Array(array=w568, index=3) -> (element=w570:dbl)
                        n372 = for {
                          N: w567 -> [_]
                          tunnel: w568 -> [w585]
                          tunnel: w570 -> [w579]
                          shift-right: [w575] -> w563
                          shift-left: dbl[][] [] ("lanes") -> [w574]
                          i -> [w584]
                          n373 = local read "lane width"() -> (w582:dbl)
                          n374 = Increment(x=w584) -> (x+1=w583:i32)
                          n375 = To Double Precision Float(number=w583) -> (double precision float=w581:dbl)
                          n376 = Multiply(x=w582, y=w581) -> (x*y=w580:dbl)
                          n377 = Add(x=w579, y=w580) -> (x+y=w578:dbl)
                          n378 = Replace Array Subset(array=w585, new element #1=w578, index #1=3 ("index"), new element #2=0.0 ("new element/subarray")) -> (w576:dbl[])  [unwired: 1 in]
                          n379 = Build Array (concatenate)(w576, w574) -> (w575:dbl[][])
                        }
                        n380 = Build Array (concatenate)(w563, w572) -> (w571:dbl[][])
                        n381 = local write "lane_seed"(w571) -> ()
                      }
                    }
                  }
                  frame False {
                    n382 = flat-sequence {
                      tunnel: w586 -> [w593]
                      frame #0 {
                        n383 = local read "lane_seed"() -> (w598:dbl[][])
                        n384 = local read "lane num"() -> (w594:i32)
                        n385 = Subtract(x=w593, y=w594) -> (x-y=w596:i32)
                        n386 = Delete From Array(array=w598, length=w596, index (row)=0) -> (array with subset deleted=w595:dbl[][])  [unwired: 1 in, 1 out]
                        n387 = local write "lane_seed"(w595) -> ()
                      }
                    }
                    n388 = disable-structure shown="Disabled" {
                      disable-tunnel: w586 -> [w587 _]
                      frame Disabled {
                        n389 = local read "lane num"() -> (w592:i32)
                        n390 = Subtract(x=w587, y=w592) -> (x-y=w590:i32)
                        n391 = local read "lanes"() -> (w588:dbl[][])
                        n392 = Delete From Array(array=w588, length=w590, index (row)=0) -> (array with subset deleted=w591:dbl[][])  [unwired: 1 in, 1 out]
                        n393 = local write "lanes"(w591) -> ()
                      }
                      frame Enabled {
                      }
                    }
                  }
                }
              }
              frame #3 {
                n394 = local read "lane_seed"() -> (w604:dbl[][])
                n395 = Array Size(array=w604) -> (size(s)=w603:i32[])
                n396 = Index Array(array=w603, index=0) -> (element=w600:i32)
                n397 = Greater?(x=w600, y=1) -> (0:w599:bool)
                n398 = case shown="False" w599 {
                  tunnel: w604 -> [_ w632]
                  frame False {
                    n399 = flat-sequence {
                      frame #0 {
                        w606 = 3.5 ("lane width")
                        n400 = local read "lane num"() -> (w605:i32)
                        n401 = local write "lane width"(w606) -> ()
                        n402 = Multiply(x=0.5, y=w606) -> (x*y=w610:dbl)
                        n403 = for {
                          N: w605 -> [_]
                          tunnel: w606 -> [w631]
                          tunnel: w610 -> [w627]
                          tunnel: [w626] -> w613 mode=indexing
                          i -> [w630]
                          n404 = To Double Precision Float(number=w630) -> (double precision float=w629:dbl)
                          n405 = Multiply(x=w631, y=w629) -> (x*y=w628:dbl)
                          n406 = Add(x=w627, y=w628) -> (x+y=w626:dbl)
                        }
                        n407 = Reverse 1D Array(array=w613) -> (reversed array=w611:dbl[])
                        n408 = Negate(x=w611) -> (-x=w612:dbl[])
                        n409 = Build Array (concatenate)(w612, w613) -> (w614:dbl[])
                        n410 = flat-sequence {
                          tunnel: [w617] -> w607
                          tunnel: w614 -> [w615]
                          tunnel: [w615] -> w608
                          frame #0 {
                            n411 = Absolute Value(x=w615) -> (abs(x)=w616:dbl[])
                            n412 = Divide(x=45.0, y=180.0) -> (x/y=w622:dbl)
                            n413 = Multiply(x=3.141592653589793, y=w622) -> (x*y=w621:dbl)
                            n414 = Tangent(1:w621) -> (0:w620:dbl)
                            n415 = Multiply(x=w616, y=w620) -> (x*y=w619:dbl[])
                            n416 = Add(x=w619, y=3.43) -> (x+y=w617:dbl[])
                          }
                        }
                        n417 = local write "seed_x"(w608) -> ()
                        n418 = local write "seed_y"(w607) -> ()
                      }
                    }
                  }
                  frame True {
                    n419 = Index Array(array=w632, index (col)=3 ("disabled index (col)")) -> (element=w637:dbl[])  [unwired: 1 in]
                    n420 = Negate(x=w637) -> (-x=w638:dbl[])
                    n421 = flat-sequence {
                      tunnel: [w652] -> w634
                      tunnel: w638 -> [w651]
                      frame #0 {
                        n422 = Absolute Value(x=w651) -> (abs(x)=w650:dbl[])
                        n423 = Divide(x=45.0, y=180.0) -> (x/y=w657:dbl)
                        n424 = Multiply(x=3.141592653589793, y=w657) -> (x*y=w656:dbl)
                        n425 = Tangent(1:w656) -> (0:w655:dbl)
                        n426 = Multiply(x=w650, y=w655) -> (x*y=w654:dbl[])
                        n427 = Add(x=w654, y=3.43) -> (x+y=w652:dbl[])
                      }
                    }
                    n428 = for {
                      tunnel: w634 -> [w640] mode=indexing
                      tunnel: w632 -> [w644] mode=indexing
                      tunnel: [w645] -> w636 mode=indexing
                      tunnel: [w640] -> w633 mode=indexing
                      n429 = Multiply(x=w640, y=w640) -> (x*y=w641:dbl)
                      n430 = Array Subset(array=w644, length=4) -> (w642:dbl[])  [unwired: 1 in]
                      n431 = Multiply(x=w640, y=w641) -> (x*y=w649:dbl)
                      n432 = Build Array(w649, w641, w640, 1.0 ("element")) -> (w647:dbl[])
                      n433 = Multiply(x=w642, y=w647) -> (x*y=w646:dbl[])
                      n434 = Add Array Elements(numeric array=w646) -> (sum=w645:dbl)
                    }
                    n435 = local write "seed_y"(w633) -> ()
                    n436 = Negate(x=w636) -> (-x=w635:dbl[])
                    n437 = local write "seed_x"(w635) -> ()
                  }
                }
              }
            }
          }
        }
        frame #11 {
          n438 = disable-structure shown="Enabled" {
            frame Disabled {
              n439 = local read "lanes"() -> (w689:dbl[][])
              n440 = feedback #1(w689) -> (w690:dbl[][])
              n441 = for {
                tunnel: w690 -> [w743] mode=indexing
                tunnel: [w739] -> w668 mode=indexing
                shift-right: [w728] -> w688
                shift-left: w689 -> [w731]
                n442 = Index Array(array=w731, index (col)=3 ("index")) -> (element=w746:dbl[])  [unwired: 1 in]
                n443 = Index Array(array=w743, index=3) -> (element=w747:dbl)
                n444 = local read "lane width"() -> (w737:dbl)
                n445 = Subtract(x=w747, y=w746) -> (x-y=w745:dbl[])
                n446 = Absolute Value(x=w745) -> (abs(x)=w744:dbl[])
                n447 = Multiply(x=0.25, y=w737) -> (x*y=w735:dbl)
                n448 = Array Max & Min(array=w744) -> (min value=w738:dbl, min index (indices)=w730:i32)  [unwired: 2 out]
                n449 = Greater?(x=w735, y=w738) -> (0:w727:bool)
                n450 = case shown="False" w727 {
                  tunnel: w731 -> [w751 w755]
                  tunnel: w730 -> [_ w754]
                  tunnel: [dbl[] [0.0, 0.0, 0.0, 0.0, 0.0] w753] -> w729
                  tunnel: [w751 w752] -> w728
                  frame False {
                  }
                  frame True {
                    n451 = Delete From Array(array=w755, index (row)=w754) -> (deleted portion=w753:dbl[], array with subset deleted=w752:dbl[][])  [unwired: 2 in]
                  }
                }
                n452 = Select(t="Numeric", s=w727, f=1.0) -> (s? t:f=w733:dbl)
                n453 = Multiply(x=w743, y=w733) -> (x*y=w740:dbl[])
                n454 = Decrement(x=w733) -> (x-1=w742:dbl)
                n455 = Multiply(x=w742, y=w729) -> (x*y=w741:dbl[])
                n456 = Subtract(x=w740, y=w741) -> (x-y=w739:dbl[])
              }
              n457 = flat-sequence {
                tunnel: w688 -> [w698]
                tunnel: [w697] -> w687
                frame #0 {
                  n458 = Index Array(array=w698, index (col)=4 ("disabled index (col)")) -> (element=w702:dbl[])  [unwired: 1 in]
                  n459 = Equal?(x=w702, y=1.0) -> (x = y?=w700:bool[])
                  n460 = for {
                    tunnel: w700 -> [w707] mode=indexing
                    shift-right: [w705] -> w697
                    shift-left: dbl[][] [] ("lanes") -> [w706]
                    tunnel: w698 -> [w704] mode=indexing
                    n461 = case shown="False" w707 {
                      tunnel: w706 -> [w708 w711]
                      tunnel: [w708 w710] -> w705
                      tunnel: w704 -> [_ w709]
                      frame False {
                      }
                      frame True {
                        n462 = Build Array (concatenate)(w711, w709) -> (w710:dbl[][])
                      }
                    }
                  }
                }
              }
              n463 = flat-sequence {
                tunnel: w668 -> [w713]
                tunnel: [w712] -> w686
                frame #0 {
                  n464 = Index Array(array=w713, index (col)=4 ("disabled index (col)")) -> (element=w717:dbl[])  [unwired: 1 in]
                  n465 = Greater?(x=w717, y=0.5) -> (0:w715:bool[])
                  n466 = for {
                    tunnel: w715 -> [w722] mode=indexing
                    shift-right: [w720] -> w712
                    shift-left: dbl[][] [] ("lanes") -> [w721]
                    tunnel: w713 -> [w719] mode=indexing
                    n467 = case shown="False" w722 {
                      tunnel: w721 -> [w723 w726]
                      tunnel: [w723 w725] -> w720
                      tunnel: w719 -> [_ w724]
                      frame False {
                      }
                      frame True {
                        n468 = Build Array (concatenate)(w726, w724) -> (w725:dbl[][])
                      }
                    }
                  }
                }
              }
              n469 = Build Array (concatenate)(w687, w686) -> (w685:dbl[][])
              n470 = Index Array(array=w685, index (col) #1=3 ("disabled index (col)"), index (col) #2=0 ("index (col)")) -> (element #1=w683:dbl[], element #2=w681:dbl[], element #3=w680:dbl[], element #4=w679:dbl[], element #5=w678:dbl[], element #6=w677:dbl[])  [unwired: 10 in]
              n471 = Build Cluster Array(w683, w681, w680, w679, w678, w677) -> (w676:cluster{dbl, dbl, dbl, dbl, dbl, dbl}[])
              n472 = Sort 1D Array(array=w676) -> (sorted array=w675:cluster{dbl, dbl, dbl, dbl, dbl, dbl}[])
              n473 = for {
                tunnel: w675 -> [w696] mode=indexing
                tunnel: [w695] -> w674 mode=indexing
                tunnel: [w694] -> w673 mode=indexing
                tunnel: [w693] -> w672 mode=indexing
                tunnel: [w692] -> w671 mode=indexing
                tunnel: [w691] -> w670 mode=indexing
                n474 = Unbundle(w696) -> (w695:dbl, w694:dbl, w693:dbl, w692:dbl, w691:dbl)  [unwired: 1 out]
              }
              n475 = Build Array(w674, w673, w672, w671, w670) -> (w669:dbl[][])
              n476 = Transpose 2D Array(2D array=w669) -> (transposed array=w664:dbl[][])
              n477 = local write "lanes"(w664) -> ()
              n478 = Index Array(array=w664, index (col)=4 ("disabled index (col)")) -> (element=w666:dbl[])  [unwired: 1 in]
              n479 = Multiply(x=w666, y=0.99) -> (x*y=w663:dbl[])
              n480 = Replace Array Subset(array=w664, new element=w663, index (col)=4 ("disabled index (col)")) -> (w661:dbl[][])  [unwired: 1 in]
              n481 = feedback-in #1(w661) -> ()
            }
            frame Enabled {
              n482 = local read "lane_seed"() -> (w791:dbl[][])
              n483 = Index Array(array=w791, index (col)=4 ("disabled index (col)")) -> (element=w789:dbl[])  [unwired: 1 in]
              n484 = Multiply(x=w789, y=0.0) -> (x*y=w787:dbl[])
              n485 = Increment(x=w787) -> (x+1=w786:dbl[])
              n486 = Replace Array Subset(array=w791, new element=w786, index (col)=4 ("disabled index (col)")) -> (w760:dbl[][])  [unwired: 1 in]
              n487 = feedback #2(w760) -> (w758:dbl[][])
              n488 = for {
                shift-right: [w807] -> w757
                shift-left: dbl[][] [] ("lanes") -> [w808]
                tunnel: w758 -> [w800] mode=indexing
                shift-right: [w799] -> w756
                shift-left: w760 -> [w802]
                n489 = Index Array(array=w802, index (col)=3 ("disabled index (col)")) -> (element=w816:dbl[])  [unwired: 1 in]
                n490 = Index Array(array=w800, index #1=3 ("index")) -> (element #1=w805:dbl, element #2=w804:dbl)  [unwired: 1 in]
                n491 = Subtract(x=w816, y=w805) -> (x-y=w815:dbl[])
                n492 = Less?(x=w804, y=0.5) -> (x < y?=w811:bool)
                n493 = Absolute Value(x=w815) -> (abs(x)=w813:dbl[])
                n494 = Array Max & Min(array=w813) -> (min value=w809:dbl, min index (indices)=w801:i32)  [unwired: 2 out]
                n495 = Greater?(x=0.5, y=w809) -> (0:w803:bool)
                n496 = Or(x=w803, y=w811) -> (x .or. y?=w810:bool)
                n497 = case shown="True" w810 {
                  tunnel: w808 -> [w821 w827]
                  tunnel: [w820 w827] -> w807
                  tunnel: w800 -> [w819 _]
                  tunnel: w803 -> [_ w826]
                  tunnel: w802 -> [w818 w825]
                  tunnel: w801 -> [_ w824]
                  tunnel: w800 -> [_ w823]
                  tunnel: [w818 w822] -> w799
                  frame False {
                    n498 = Build Array (concatenate)(w821, w819) -> (w820:dbl[][])
                  }
                  frame True {
                    n499 = case shown="True" w826 {
                      tunnel: w825 -> [w828 w838]
                      tunnel: w824 -> [_ w837]
                      tunnel: w823 -> [_ w832]
                      tunnel: [w828 w836] -> w822
                      frame False {
                      }
                      frame True {
                        w834 = 0.2
                        n500 = Index Array(array=w838, index (row)=w837) -> (element=w835:dbl[])  [unwired: 1 in]
                        n501 = Multiply(x=w835, y=w834) -> (x*y=w830:dbl[])
                        n502 = Decrement(x=w834) -> (x-1=w833:dbl)
                        n503 = Multiply(x=w833, y=w832) -> (x*y=w831:dbl[])
                        n504 = Subtract(x=w830, y=w831) -> (x-y=w829:dbl[])
                        n505 = Replace Array Subset(array=w838, new element=w829, index (row)=w837) -> (w836:dbl[][])  [unwired: 1 in]
                      }
                    }
                  }
                }
              }
              n506 = Index Array(array=w757, index (col)=4 ("disabled index (col)")) -> (element=w782:dbl[])  [unwired: 1 in]
              n507 = Multiply(x=w782, y=0.9) -> (x*y=w780:dbl[])
              n508 = Replace Array Subset(array=w757, new element=w780, index (col)=4 ("disabled index (col)")) -> (w779:dbl[][])  [unwired: 1 in]
              n509 = Build Array (concatenate)(w756, w779) -> (w763:dbl[][])
              n510 = Index Array(array=w763, index (col) #1=3 ("disabled index (col)"), index (col) #2=0 ("index (col)")) -> (element #1=w777:dbl[], element #2=w775:dbl[], element #3=w774:dbl[], element #4=w773:dbl[], element #5=w772:dbl[], element #6=w771:dbl[])  [unwired: 10 in]
              n511 = Build Cluster Array(w777, w775, w774, w773, w772, w771) -> (w770:cluster{dbl, dbl, dbl, dbl, dbl, dbl}[])
              n512 = Sort 1D Array(array=w770) -> (sorted array=w762:cluster{dbl, dbl, dbl, dbl, dbl, dbl}[])
              n513 = Reverse 1D Array(array=w762) -> (reversed array=w761:cluster{dbl, dbl, dbl, dbl, dbl, dbl}[])
              n514 = for {
                tunnel: w761 -> [w798] mode=indexing
                tunnel: [w797] -> w769 mode=indexing
                tunnel: [w796] -> w768 mode=indexing
                tunnel: [w795] -> w767 mode=indexing
                tunnel: [w794] -> w766 mode=indexing
                tunnel: [w793] -> w765 mode=indexing
                n515 = Unbundle(w798) -> (w797:dbl, w796:dbl, w795:dbl, w794:dbl, w793:dbl)  [unwired: 1 out]
              }
              n516 = Build Array(w769, w768, w767, w766, w765) -> (w764:dbl[][])
              n517 = Transpose 2D Array(2D array=w764) -> (transposed array=w792:dbl[][])
              n518 = feedback-in #2(w792) -> ()
              n519 = local write "lanes"(w792) -> ()
            }
            frame Disabled {
            }
          }
        }
      }
    }
    frame #2 {
      n520 = Tick Count (ms)() -> (millisecond timer value=w841:u32)
      n521 = Subtract(x=w841, y=w840) -> (x-y=→"time":u32)
    }
    frame #3 {
      n522 = local read "seed_y"() -> (w856:dbl[])
      n523 = local read "seed_x"() -> (w863:dbl[])
      n524 = flat-sequence {
        tunnel: [w866] -> w848
        tunnel: [w868] -> w847
        tunnel: w848 -> [w867]
        frame #0 {
          n525 = local read "lanes"() -> (w866:dbl[][])
        }
        frame #1 {
          n526 = for {
            tunnel: [w871] -> w868 mode=indexing
            tunnel: w867 -> [w869] mode=indexing
            n527 = local read "lane_x"() -> (w880:dbl[])
            n528 = Index Array(array=w869, index #1=0 ("index")) -> (element #1=w877:dbl, element #2=w876:dbl, element #3=w875:dbl, element #4=w870:dbl)  [unwired: 3 in]
            n529 = Multiply(x=w880, y=w875) -> (x*y=w872:dbl[])
            n530 = Multiply(x=w880, y=w880) -> (x*y=w879:dbl[])
            n531 = Multiply(x=w880, y=w879) -> (x*y=w878:dbl[])
            n532 = Multiply(x=w879, y=w876) -> (x*y=w873:dbl[])
            n533 = Multiply(x=w878, y=w877) -> (x*y=w874:dbl[])
            n534 = Compound Arithmetic op=ADD(w874, w873, w872, w870) -> (w871:dbl[])
          }
        }
      }
      n535 = local read "lanes"() -> (w845:dbl[][])
      n536 = local read "sensors"() -> (w843:dbl[][])
      n537 = local read "sensors"() -> (w842:dbl[][])
      n538 = for {
        tunnel: w845 -> [_] mode=indexing
        tunnel: [w865] -> w844 mode=indexing
        n539 = local read "lane_x"() -> (w865:dbl[])
      }
      n540 = Negate(x=w863) -> (-x=w864:dbl[])
      n541 = call "Convert to Dynamic Data4"("Array"=w856) -> ("Dynamic Data Type"=w857:dynamicdata)  [unwired: 3 in]
      n542 = call "Convert to Dynamic Data3"("Array"=w864) -> ("Dynamic Data Type"=w855:dynamicdata)  [unwired: 3 in]
      n543 = Index Array(array=w843, index (col)=1 ("disabled index (col)")) -> (element=w852:dbl[])  [unwired: 1 in]
      n544 = Index Array(array=w842, index (col)=0 ("disabled index (col)")) -> (element=w861:dbl[])  [unwired: 1 in]
      n545 = Negate(x=w861) -> (-x=w862:dbl[])
      n546 = call "Convert to Dynamic Data2"("Array"=w852) -> ("Dynamic Data Type"=w853:dynamicdata)  [unwired: 3 in]
      n547 = call "Convert to Dynamic Data5"("2D Array"=w844) -> ("Dynamic Data Type"=w849:dynamicdata)  [unwired: 3 in]
      n548 = call "Convert to Dynamic Data"("Array"=w862) -> ("Dynamic Data Type"=w851:dynamicdata)  [unwired: 3 in]
      n549 = Merge Signals(w853, w857, w849) -> (w859:dynamicdata)
      n550 = call "Convert to Dynamic Data6"("2D Array"=w847) -> ("Dynamic Data Type"=w846:dynamicdata)  [unwired: 3 in]
      n551 = Merge Signals(w851, w855, w846) -> (w860:dynamicdata)
      n552 = call "Build XY Graph"("Y Input"=w860, "X Input"=w859) -> ("XY Graph"=→"XY Graph":cluster{"Y":dbl[], "Y":dbl[]}[])  [unwired: 3 in, 6 out]
    }
  }
